vi "EncoderB(D0BD).vi"() -> ()   [LabVIEW 2021]
uses:
  BISS_1SL_interface_7.7.0/lv_interface/enum/BISS_InterfaceEnum.ctl
  BISS_1SL_interface_7.7.0/lv_interface/enum/BISS_InterfaceInfoEnum.ctl
  BISS_1SL_interface_7.7.0/lv_interface/enum/BISS_ComParamEnum.ctl
  BISS_1SL_interface_7.7.0/lv_interface/enum/BISS_FrameParamEnum.ctl
  BISS_1SL_interface_7.7.0/lv_interface/enum/BISS_EdsParamEnum.ctl
  BISS_1SL_interface_7.7.0/lv_interface/enum/BISS_ErrorTypeEnum.ctl
  BISS_1SL_interface_7.7.0/lv_interface/dll_demo/BiSS Interface Demo Functions.ctl
  BISS_1SL_interface_7.7.0/lv_interface/BISS1SL_Interface.lvlib
panel:
  in  "Stop Button":bool
  in  "TabControl":T1(tab)
  in  "BISS_InterfaceInfoEnum":T2 format="0x%02x"
  out "BISS_InterfaceEnum":T3 format="0x%02x"
  in  "BISS_InterfaceEnum":T3=enum."BISS_MB5U" format="0x%02x"
  in  "Close":bool caption="BiSS_Close"
  in  "Get Interface":bool caption="BiSS_GetInterface"
  in  "Set Interface":bool caption="BiSS_SetInterface"
  in  "Open":bool caption="BiSS_Open"
  in  "pcInterfaceOption":string="D0BD"
  in  "Get Interface Info":bool caption="BiSS_GetInterfaceInfo"
  out "pcInterfaceInfo":string
  in  "Write Master Params":bool caption="BiSS_WriteMasterParams"
  in  "pcFilename":path
  in  "Load DLL Config":bool caption="BiSS_LoadDLLConfig"
  in  "pcFilename 2":path=path "C:/Users/TSSW/Documents/Kenneth Feb/BISS Test Vi/BiSS_config.cfg"
  in  "Save DLL Config":bool caption="BiSS_SaveDLLConfig"
  in  "Get Slave Label":bool caption="BiSS_GetSlaveLabel"
  in  "ulSlave 2":u32 format="%.0x"
  out "pcCompleteLabel 2":string
  out "pcSlaveLabel 2":string
  out "pcManufacturerLabel 2":string
  in  "Set FTDI Freq":bool caption="BiSS_SetFTDIFreq"
  in  "ulFreqL":u32=4 format="%0x"
  in  "ulFreqH":u32=4 format="%0x"
  out "Displacement vs Time":waveform(sgl)(graph)
  out "pulValues":u64[](array[numeric]) format="%.0x"
  in  "ulCycleCount":u32 format="%.0x"
  in  "ulContentIndex":u32 format="%.0x"
  in  "ulDataChannel":u32 format="%.0x"
  in  "Get SCD Frame Content Ex":bool caption="BiSS_GetScdFrameContentEx"
  in  "Read SCD Frames":bool caption="BiSS_ReadScdFrames"
  in  "ulCycleCnt":u32=1 format="%.0x"
  out "pulDataScdH":u32[](array[numeric]) format="%.0x"
  out "pulDataScdL":sgl[](array[numeric]) format="%#_8g mm"
  out "pulStatus":u32[](array[numeric]) format="%.0x"
  out "pulTimestamp":u32[](array[numeric]) format="%.0x"
  in  "Get SCD Frame":bool caption="BiSS_GetScdFrame"
  in  "ulFrameIndex":u32 format="%.0x"
  out "pulDataScdH":u32[](array[numeric]) format="%.0x"
  out "pulDataScdL":u32[](array[numeric]) format="%.0x"
  out "pulStatus":u32 format="%.0x"
  out "pulTimestamp":u32 format="%.0x"
  in  "ulDataChannel":u32 format="%.0x"
  in  "Get SCD Frame Ex":bool caption="BiSS_GetScdFrameEx"
  in  "ulCycleCount":u32 format="%.0x"
  out "pulTimestamp":u32[](array[numeric]) format="%.0x"
  out "pulDataScdH":u32[](array[numeric]) format="%.0x"
  out "pulDataScdL":u32[](array[numeric]) format="%.0x"
  out "pulStatus":u32[](array[numeric]) format="%.0x"
  in  "Get SCD Frame Content":bool caption="BiSS_GetScdFrameContent"
  in  "ulDataChannel":u32 format="%.0x"
  in  "ulContentIndex":u32 format="%.0x"
  out "pulValues":u32[](array[numeric]) format="%.0x"
  in  "ulCycleCount":u32 format="%.0x"
  in  "stop":bool
  out "Loop Time [ms]":u32
  in  "Update Time [ms]":u32=1000
  out "BISS_ErrorTypeEnum":T4 format="0x%02x"
  in  "Get DLL Version":bool caption="BiSS_GetDLLVersion"
  out "pulDllVersion":u32[](array[numeric]) format="%.0x"
  in  "Calculate CRC":bool caption="BiSS_CalculateCRC"
  in  "ulCrcPoly":u32 format="%.0x"
  in  "pulData":u32[](array[numeric]) format="%.0x"
  in  "ulByteCount":u32 format="%.0x"
  out "pulCheckSum":u32 format="%.0x"
  in  "Calculate CRC Ex":bool caption="BiSS_CalculateCRCEx"
  out "pulCheckSum":u32 format="%.0x"
  in  "ulByteCount":u32 format="%.0x"
  in  "pulData":u32[](array[numeric]) format="%.0x"
  in  "ulCrcPoly":u32 format="%.0x"
  in  "ulCRCStartValue":u32 format="%.0x"
  in  "Get Last Error":bool caption="BiSS_GetLastError"
  out "pulLastError":u32 format="%0x"
  out "pcErrorText":string
  in  "Get MB3U Pins":bool caption="BiSS_GetMB3UPins"
  out "pulDir":u32 format="%.0x"
  out "pulValue":u32 format="%.0x"
  in  "ulDir":u32 format="%.0x"
  in  "Set MB3U Pins":bool caption="BiSS_SetMB3UPins"
  in  "ulValue":u32 format="%.0x"
  in  "Set Slave Label":bool caption="BiSS_SetSlaveLabel"
  in  "ulSlave":u32 format="%.0x"
  in  "pcSlaveLabel":string
  in  "pcManufacturerLabel":string
  in  "pcCompleteLabel":string
  in  "Set SCD Content Labels":bool caption="BiSS_SetScdContentLabels"
  in  "ulDataChannel":u32 format="%.0x"
  in  "ulContentIndex":u32 format="%.0x"
  in  "pcScdContentLabel":string
  in  "pcScdContentUnit":string
  in  "Get SCD Content Labels":bool caption="BiSS_GetScdContentLabels"
  in  "ulDataChannel":u32 format="%.0x"
  in  "ulContentIndex":u32 format="%.0x"
  out "pcSCDContentLabel":string
  out "pcSCDContentUnit":string
  in  "BISS_FrameParamEnum":T5 format="0x%02x"
  in  "BISS_FrameParamEnum":T5 format="0x%02x"
  in  "BISS_ComParamEnum":T6 format="0x%02x"
  in  "BISS_ComParamEnum":T6 format="0x%02x"
  in  "pcFilename":path
  in  "Set Com Param":bool caption="BiSS_SetComParam"
  in  "Auto Detection":bool caption="BiSS_Autodetection"
  in  "ulWriteMasterParams":u32 format="%.0x"
  out "pulSlaveCount":u32 format="%.0x"
  in  "ulValue":u32 format="%.0x"
  in  "Get Com Param":bool caption="BiSS_GetComParam"
  out "pulValue":u32 format="%.0x"
  in  "Set Frame Param":bool caption="BiSS_FrameParamEnum"
  in  "ulDataChannel":u32 format="%.0x"
  in  "ulValue":u32 format="%.0x"
  in  "Get Frame Param":bool caption="BiSS_GetFrameParam"
  out "pulValue":u32 format="%.0x"
  in  "ulDataChannel":u32 format="%.0x"
  in  "Init BiSS Comm":bool caption="BiSS_InitBissComm"
  in  "Write Slave Register":bool caption="BiSS_WriteSlaveRegister"
  in  "ulProtocol":u32 format="%.0x"
  in  "ulSlaveId":u32 format="%.0x"
  in  "ulRegisterAddress":u32 format="%.0x"
  in  "pulRegisterContent":u32[](array[numeric]) format="%.0x"
  in  "pulNumberOfBytes":u32 format="%.0x"
  in  "Read Slave Register":bool caption="BiSS_ReadSlaveRegister"
  in  "ulProtocol":u32 format="%.0x"
  in  "ulSlaveId":u32 format="%.0x"
  in  "ulRegisterAddress":u32 format="%.0x"
  in  "pulNumberOfBytes":u32 format="%.0x"
  out "pulRegisterContent":u32[](array[numeric]) format="%.0x"
  in  "Read SCD":bool caption="BiSS_ReadSCD"
  in  "ulStartControlFrame":u32 format="%.0x"
  out "pulScdValid":u32 format="%.0x"
  out "pulControlFrameEnd":u32 format="%.0x"
  out "pulDataScdH":u32[](array[numeric]) format="%.0x"
  out "pulDataScdL":u32[](array[numeric]) format="%.0x"
  in  "ulIds":u32 format="%.0x"
  in  "ulCmd":u32 format="%.0x"
  in  "Send Command":bool caption="BiSS_SendCommand"
  in  "Get SCD Content":bool caption="BiSS_GetScdContent"
  in  "ulDataChannel":u32 format="%.0x"
  out "pulScdContentValues":u32[](array[numeric]) format="%.0x"
  in  "Get SCD Content Ex":bool caption="BiSS_GetScdContentEx"
  in  "ulDataChannel":u32 format="%.0x"
  out "pulScdContentValues":u64[](array[numeric]) format="%.0x"
  in  "Set SCD Content Params":bool caption="BiSS_SetScdContentParams"
  in  "ulDataChannel":u32 format="%.0x"
  in  "ulContentIndex":u32 format="%.0x"
  in  "pScdContentItems":T7 {"lOffset" format="%.0x"; "ulResolution" format="%.0x"; "ulDataLength" format="%.0x"; "ulZero" format="%.0x"}
  in  "Get SCD Content Params":bool caption="BiSS_GetScdContentParams"
  in  "ulDataChannel":u32 format="%.0x"
  in  "ulContentIndex":u32 format="%.0x"
  out "pScdContentItems":T7 {"ulZero" format="%.0x"; "ulDataLength" format="%.0x"; "ulResolution" format="%.0x"; "lOffset" format="%.0x"}
  in  "BISS_EdsParamEnum":T8 format="0x%02x"
  in  "BISS_EdsParamEnum":T8 format="0x%02x"
  in  "Set EDS Param":bool caption="BiSS_SetEdsParam"
  in  "ulValue":u32 format="%.0x"
  out "pulValue":u32 format="%.0x"
  in  "Get EDS Param":bool caption="BiSS_GetEdsParam"
  in  "Set EDS Register":bool caption="BiSS_SetEdsRegister"
  in  "ulAdr":u32 format="%.0x"
  in  "ulValue":u32 format="%.0x"
  in  "Get EDS Register":bool caption="BiSS_GetEdsRegister"
  in  "ulAdr":u32 format="%.0x"
  out "pulValue":u32 format="%.0x"
  in  "Read EDS Params":bool caption="BiSS_ReadEdsParams"
  in  "ulSlaveId":u32 format="%.0x"
  in  "Write EDS Params":bool caption="BiSS_WriteEdsParams"
  in  "ulSlaveId":u32 format="%.0x"
  in  "pcFilename":path
  in  "Write Master Register":bool caption="BiSS_ WriteMasterRegister"
  in  "ulRegisterAddress":u32 format="%.0x"
  in  "ulRegisterContent":u32 format="%.0x"
  in  "Read Master Register":bool caption="BiSS_ ReadMasterRegister"
  in  "ulRegisterAddress":u32 format="%.0x"
  out "pulRegisterContent":u32 format="%.0x"
  in  "Get Master Register":bool caption="BiSS_ GetMasterRegister"
  in  "ulRegisterAddress":u32 format="%.0x"
  out "pulRegisterContent":u32 format="%.0x"
  in  "Save Master Config":bool caption="BiSS_ SaveMasterConfig"
  in  "pcFilename":path
  in  "Save Register":bool caption="BiSS_ SaveRegister"
  in  "pcFilename":path
  in  "ulStartAdr":u32 format="%.0x"
  in  "ulNumberOfBytes":u32 format="%.0x"
  in  "pulData":u32[](array[numeric]) format="%.0x"
  in  "Load Register":bool caption="BiSS_ LoadRegister"
  in  "ulStartAdr":u32 format="%.0x"
  in  "ulNumberOfBytes":u32 format="%.0x"
  out "pulData":u32[](array[numeric]) format="%.0x"
  # "BiSS Interface Library Demo"
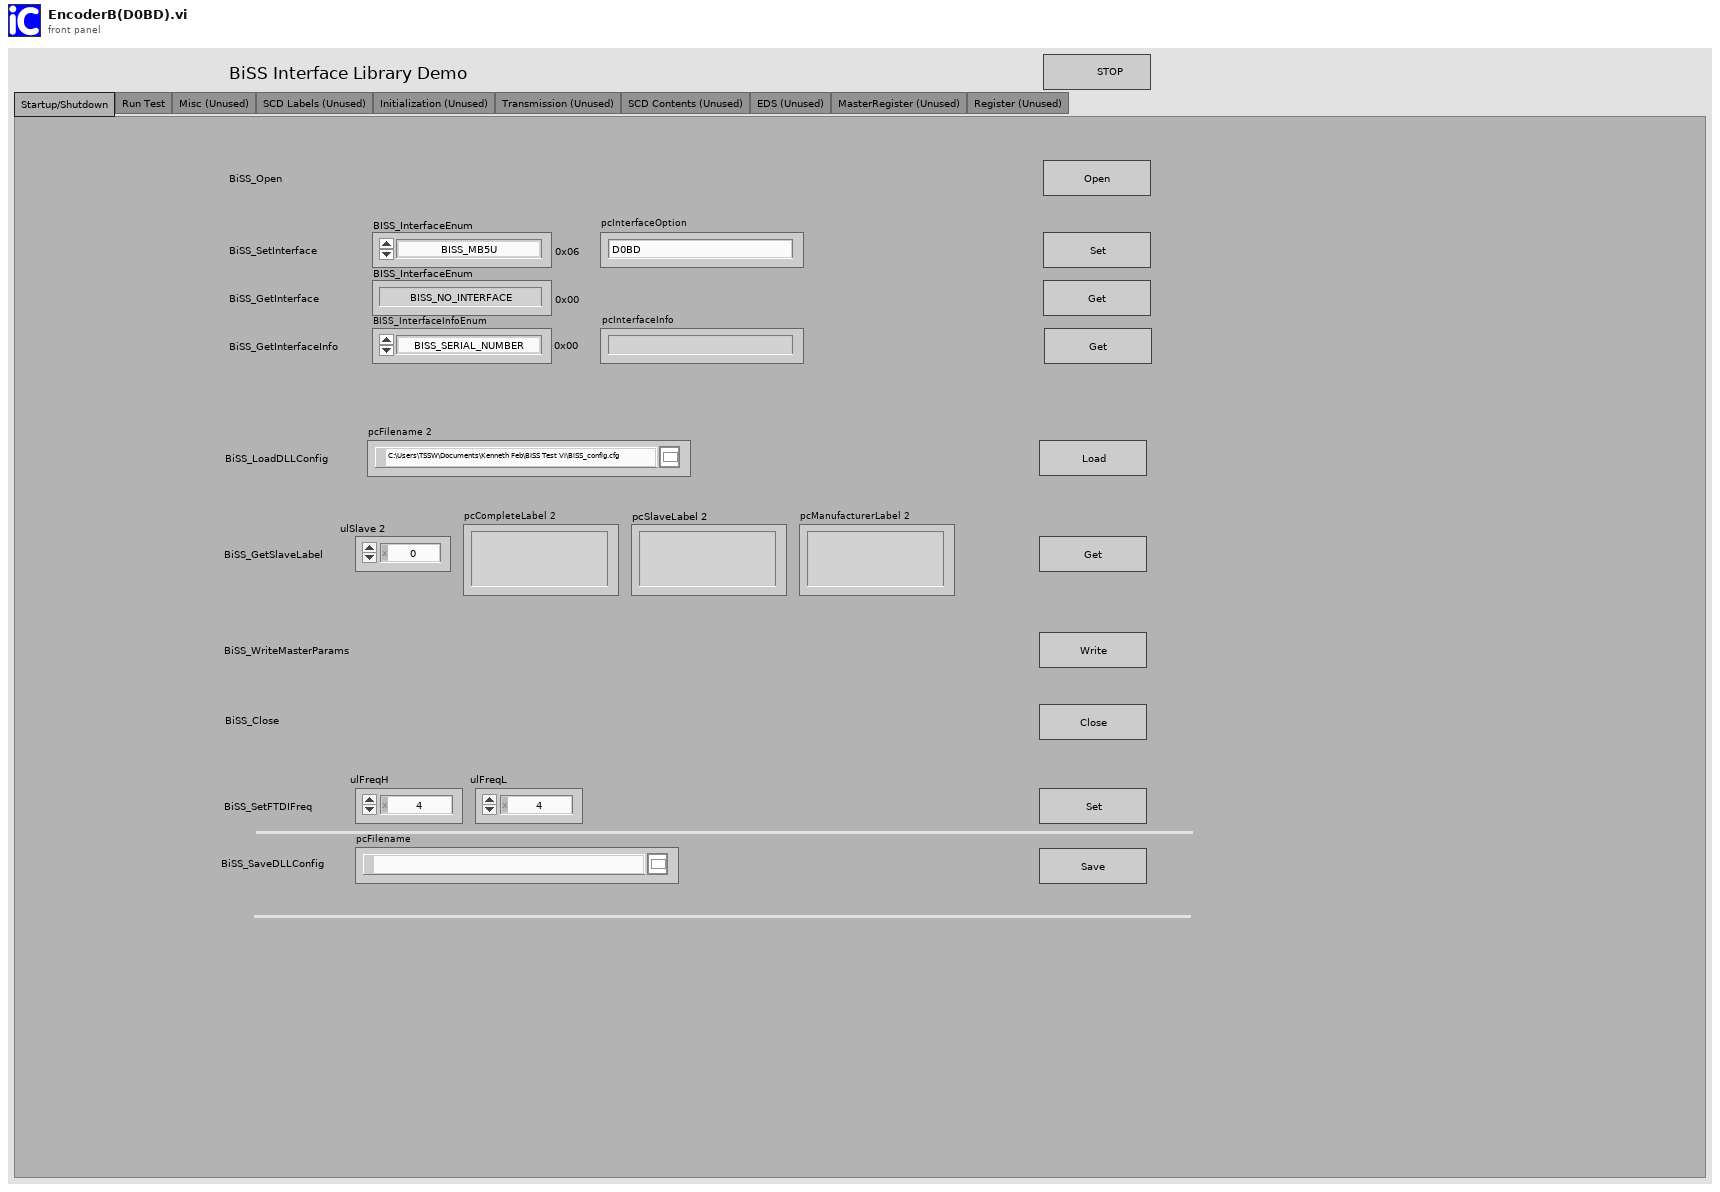
[diagram p1: front panel]
types:
  T1 = enum32{"Startup/Shutdown", "Run Test", "Misc (Unused)", "SCD Labels (Unused)", "Initialization (Unused)", "Transmission (Unused)", "SCD Contents (Unused)", "EDS (Unused)", "MasterRegister (Unused)", "Register (Unused)"}
  T2 = typedef "BISS1SL_Interface.lvlib/BISS_InterfaceInfoEnum.ctl" = enum32{"BISS_SERIAL_NUMBER", "BISS_DRIVER_VERSION"}
  T3 = typedef "BISS1SL_Interface.lvlib/BISS_InterfaceEnum.ctl" = enum32{"BISS_NO_INTERFACE", "BISS_MB3D_INT", "BISS_MB3D_MOT", "BISS_MB3A", "BISS_MB3U", "BISS_MB4U", "BISS_MB5U", "BISS_MB3U_SPI"}
  T4 = typedef "BISS1SL_Interface.lvlib/BISS_ErrorTypeEnum.ctl" = enum32{"BISS_NONE", "BISS_HINT", "BISS_WARNING", "BISS_PROGRAMMING_ERROR", "BISS_OPERATING_ERROR", "BISS_COMMUNICATION_ERROR"}
  T5 = typedef "BISS1SL_Interface.lvlib/BISS_FrameParamEnum.ctl" = enum32{"BISS_SCD_LENGTH", "BISS_SCD_CRC_POLY", "BISS_SCD_CRC_INVERT", "BISS_SCD_CONTENT_COUNT", "BISS_RESERVED", "BISS_SLAVEID", "BISS_IDCOUNT", "BISS_CRCS", "BISS_GRAYS", "BISS_GRAY_MSB", "BISS_GRAY_LSB", "BISS_CRC_CLOSING_VALUE"}
  T6 = typedef "BISS1SL_Interface.lvlib/BISS_ComParamEnum.ctl" = enum32{"BISS_MASTER_VERSION", "BISS_MASTER_REVISION", "BISS_PROTOCOL", "BISS_CLKENI", "BISS_FREQ_SCD", "BISS_FREQ_REG", "BISS_FREQ_AGS", "BISS_SLAVE_ID", "BISS_REGISTER_ADDRESS", "BISS_WNR", "BISS_REGISTER_VALUE", "BISS_SSIWRITE", "BISS_SSIWRITE_TIMEOUT", "BISS_MAX_DATACH_CNT", "BISS_MAX_REG_CNT", "BISS_EN_MO", "BISS_FREQ_AGS_REG", "BISS_EDS_BANK", "BISS_DISABLE_TIMEOUT", "BISS_ENABLE_TTL", "BISS_NUMBER_OF_DATA_CHANNELS", "BISS_SSIWRITE_DL", "BISS_SLAVELOC"}
  T7 = cluster{"ulZero":u32, "ulDataLength":u32, "ulResolution":u32, "lOffset":i32}
  T8 = typedef "BISS1SL_Interface.lvlib/BISS_EdsParamEnum.ctl" = enum32{"BISS_EDS_EDS_VER", "BISS_EDS_EDS_LEN", "BISS_EDS_USR_STA", "BISS_EDS_USR_END", "BISS_EDS_TMA", "BISS_EDS_TO_MIN", "BISS_EDS_TO_MAX", "BISS_EDS_TOS_MIN", "BISS_EDS_TOS_MAX", "BISS_EDS_TCLK_MIN", "BISS_EDS_TCLK_MAX", "BISS_EDS_TCYC", "BISS_EDS_TBUSY_S", "BISS_EDS_BUSY_S", "BISS_EDS_PON_DLY", "BISS_EDS_DC_NUM", "BISS_EDS_SL_NUM", "BISS_EDS_SL_OFF", "BISS_EDS_BANK1", "BISS_EDS_DLEN1", "BISS_EDS_FORMAT1_STOP", "BISS_EDS_FORMAT1_ALIGN", "BISS_EDS_FORMAT1_TYPE", "BISS_EDS_CPOLY1", "BISS_EDS_BANK2", "BISS_EDS_DLEN2", "BISS_EDS_FORMAT2_STOP", "BISS_EDS_FORMAT2_ALIGN", "BISS_EDS_FORMAT2_TYPE", "BISS_EDS_CPOLY2", "BISS_EDS_BANK3", "BISS_EDS_DLEN3", "BISS_EDS_FORMAT3_STOP", "BISS_EDS_FORMAT3_ALIGN", "BISS_EDS_FORMAT3_TYPE", "BISS_EDS_CPOLY3", "BISS_EDS_BANK4", "BISS_EDS_DLEN4", "BISS_EDS_FORMAT4_STOP", "BISS_EDS_FORMAT4_ALIGN", "BISS_EDS_FORMAT4_TYPE", "BISS_EDS_CPOLY4", "BISS_EDS_BANK5", "BISS_EDS_DLEN5", "BISS_EDS_FORMAT5_STOP", "BISS_EDS_FORMAT5_ALIGN", "BISS_EDS_FORMAT5_TYPE", "BISS_EDS_CPOLY5", "BISS_EDS_BANK6", "BISS_EDS_DLEN6", "BISS_EDS_FORMAT6_STOP", "BISS_EDS_FORMAT6_ALIGN", "BISS_EDS_FORMAT6_TYPE", "BISS_EDS_CPOLY6", "BISS_EDS_BANK7", "BISS_EDS_DLEN7", "BISS_EDS_FORMAT7_STOP", "BISS_EDS_FORMAT7_ALIGN", "BISS_EDS_FORMAT7_TYPE", "BISS_EDS_CPOLY7", "BISS_EDS_BANK8", "BISS_EDS_DLEN8", "BISS_EDS_FORMAT8_STOP", "BISS_EDS_FORMAT8_ALIGN", "BISS_EDS_FORMAT8_TYPE", "BISS_EDS_CPOLY8", "BISS_EDS_BC_OFF", "BISS_EDS_BP_VER", "BISS_EDS_BP_LEN", "BISS_EDS_BP_ID", "BISS_EDS_FB1", "BISS_EDS_FB2", "BISS_EDS_PON_PDL", "BISS_EDS_EN_TYP", "BISS_EDS_POS_NUM", "BISS_EDS_MT_LEN", "BISS_EDS_MT_FMT", "BISS_EDS_CO_LEN", "BISS_EDS_CO_FMT", "BISS_EDS_FI_LEN", "BISS_EDS_FI_FMT", "BISS_EDS_MT_CNT", "BISS_EDS_SIP_CNT", "BISS_EDS_SIP_RES", "BISS_EDS_CPOLY", "BISS_EDS_CSTART", "BISS_EDS_ABS_ACU", "BISS_EDS_REL_ACU", "BISS_EDS_SPD_ACU", "BISS_EDS_HYST", "BISS_EDS_SPD_MAX", "BISS_EDS_ACC_MAX", "BISS_EDS_TMP_MIN", "BISS_EDS_TMP_MAX", "BISS_EDS_VLT_MIN", "BISS_EDS_VLT_MAX", "BISS_EDS_CUR_MAX"}
  T9 = typedef "BiSS Interface Demo Functions.ctl" = enum16{"Start Demo", "Open", "Close", "Set Interface", "Set Interface 2", "Get Interface", "Get Interface 2", "Get Interface Info", "Get Interface Info 2", "Auto Detection", "Set Com Param", "Get Com Param", "Set Frame Param", "Get Frame Param", "Write Master Params", "Set FTDI Freq", "Init BiSS Comm", "Write Slave Register", "Read Slave Register", "Read SCD", "Send Command", "Set Slave Label", "Get Slave Label", "Set SCD Content Labels", "Get SCD Content Labels", "Get SCD Content", "Get SCD Content Ex", "Set SCD Content Params", "Get SCD Content Params", "Read SCD Frames", "Get SCD Frame", "Get SCD Frame Ex", "Get SCD Frame Content", "Get SCD Frame Content Ex", "Set EDS Param", "Get EDS Param", "Set EDS Register", "Get EDS Register", "Read EDS Params", "Write EDS Params", "Get DLL Version", "Calculate CRC", "Calculate CRC Ex", "Save DLL Config", "Load DLL Config", "Get Last Error", "Get MB3U Pins", "Set MB3U Pins", "Write Master Register", "Read Master Register", "Get Master Register", "Save Master Config", "Save Register", "Load Register", "Stop Demo"}
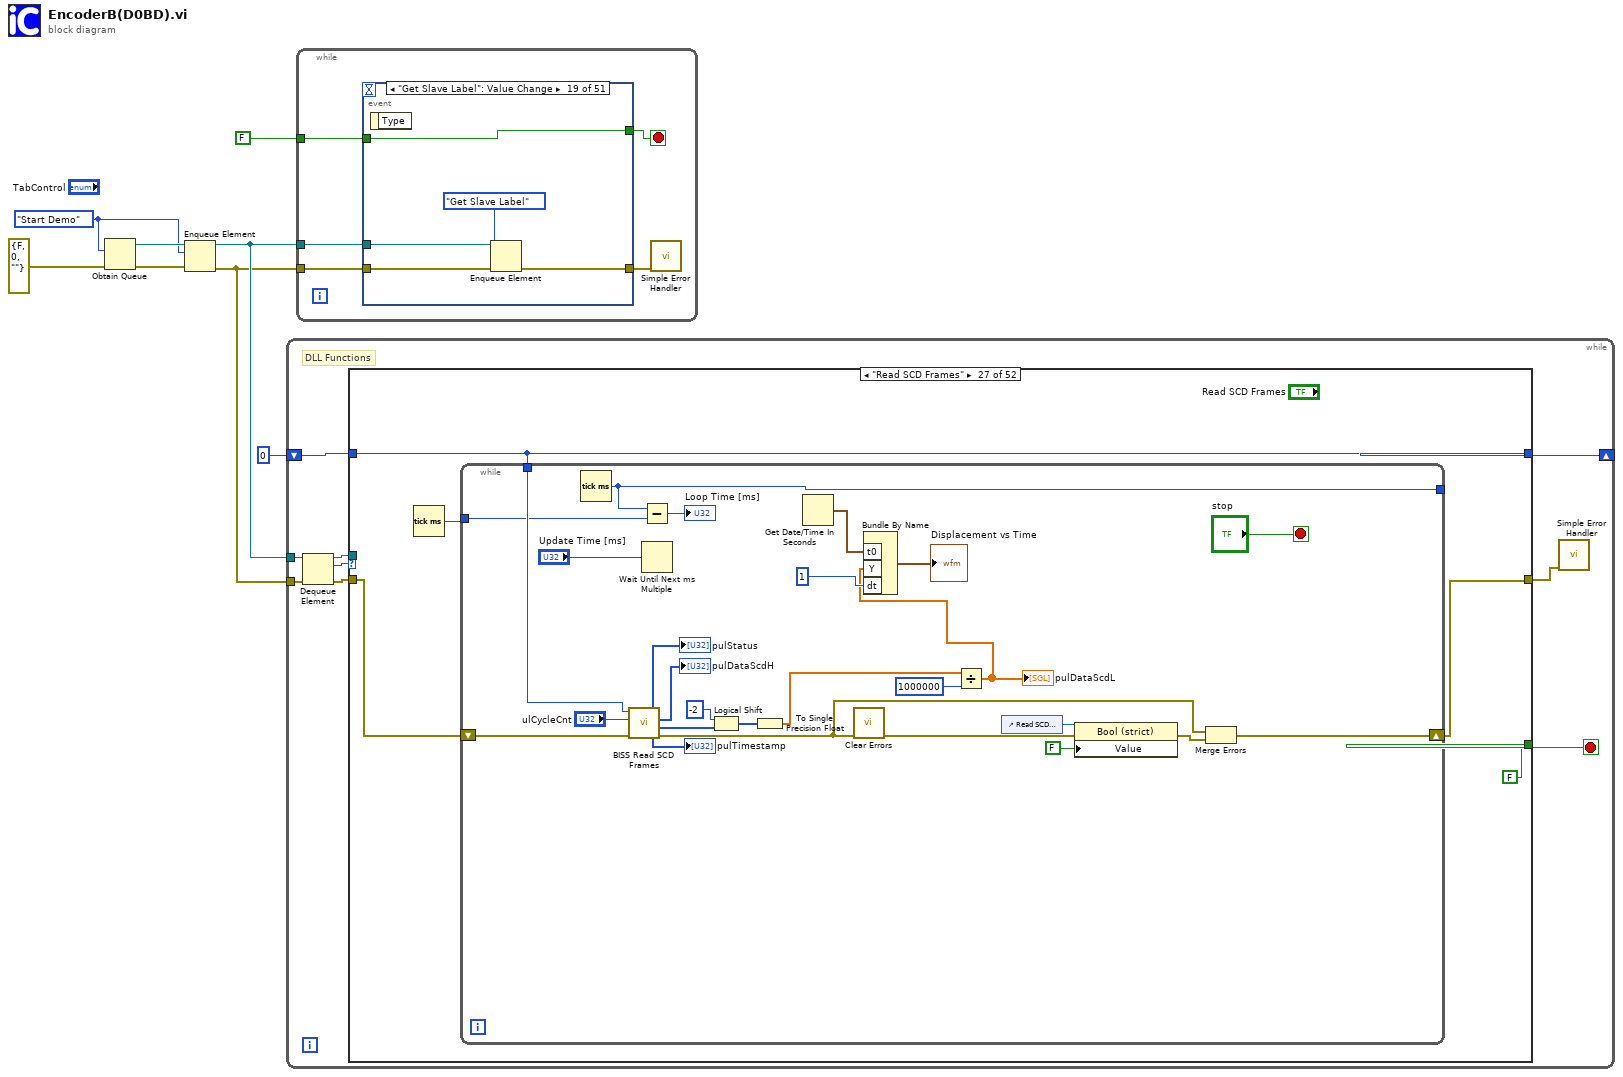
[diagram p0: block diagram]
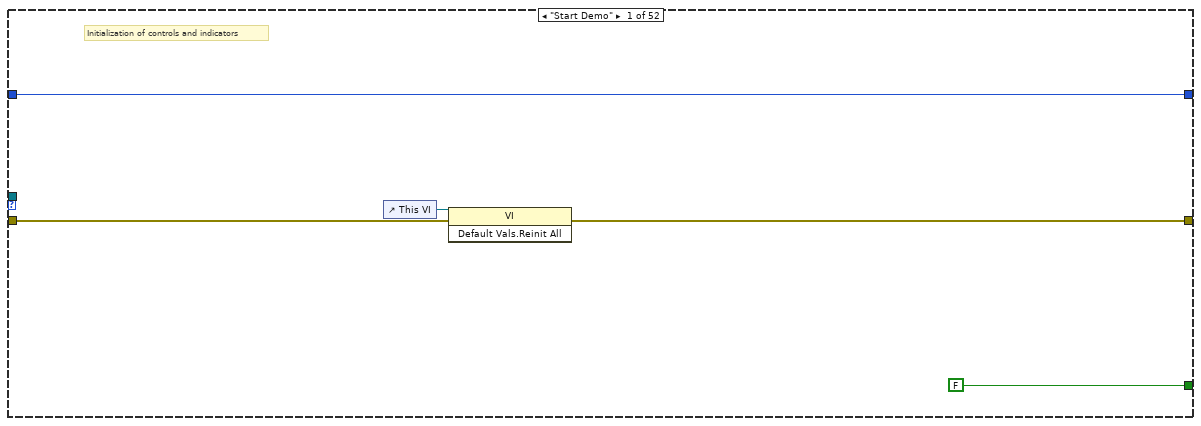
[diagram p2: hidden frame]
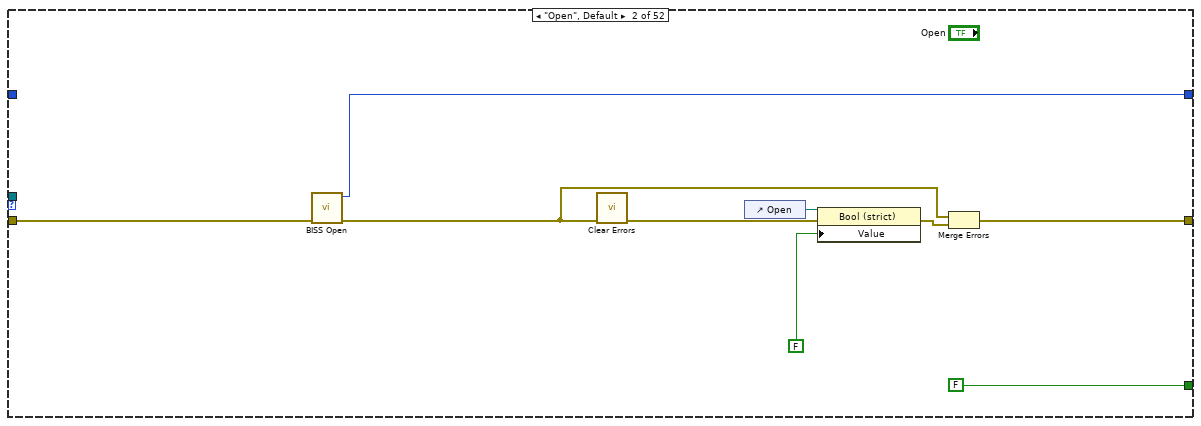
[diagram p3: hidden frame]
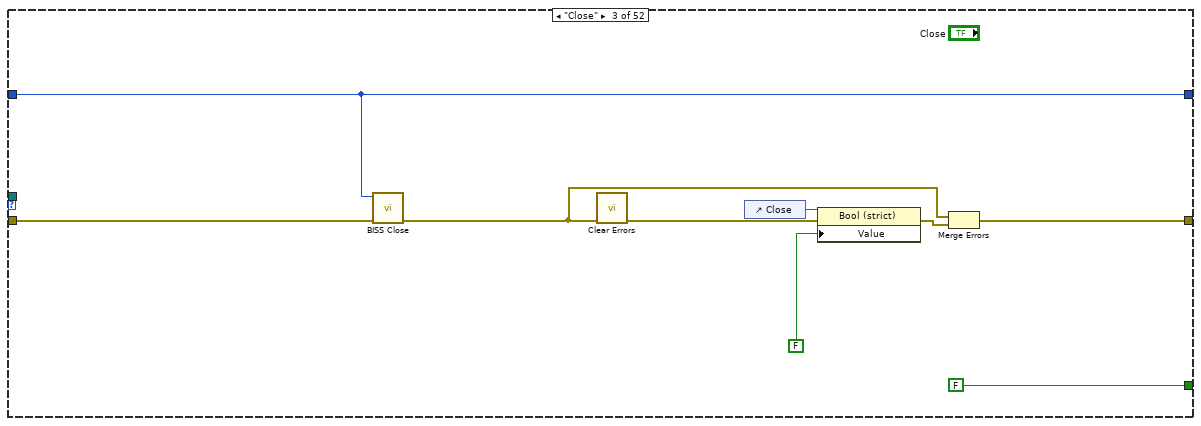
[diagram p4: hidden frame]
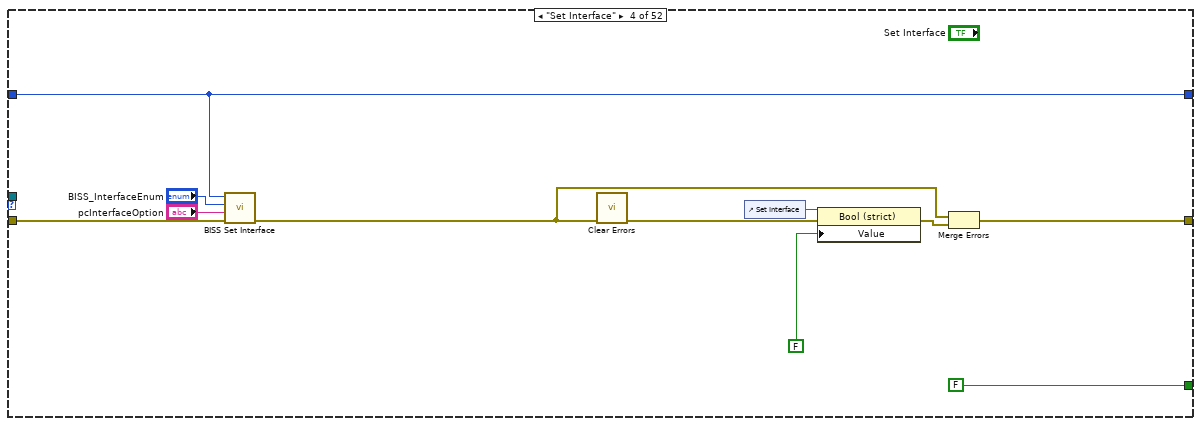
[diagram p5: hidden frame]
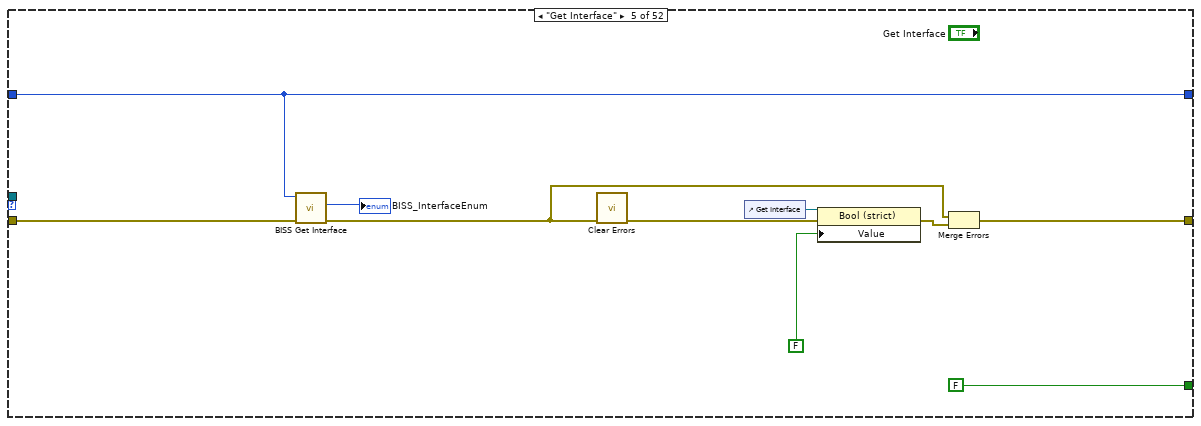
[diagram p6: hidden frame]
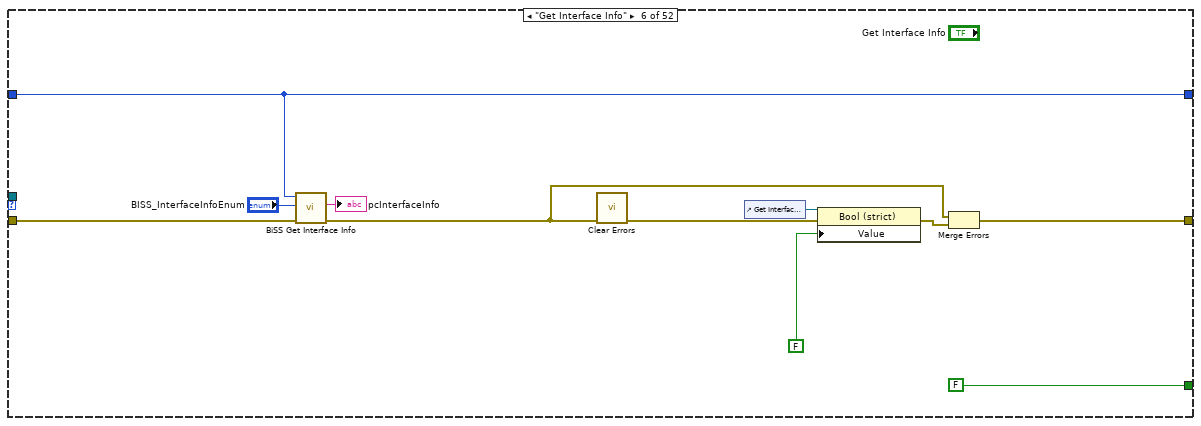
[diagram p7: hidden frame]
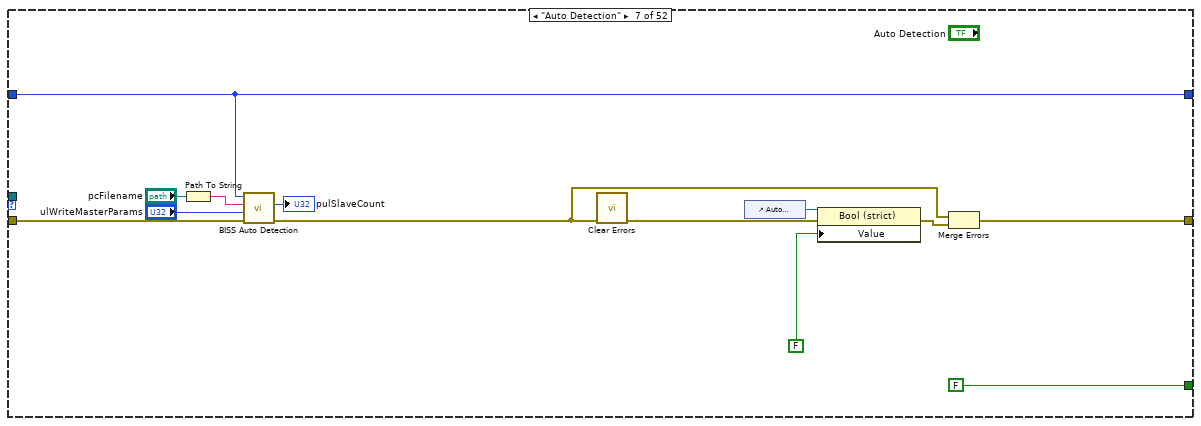
[diagram p8: hidden frame]
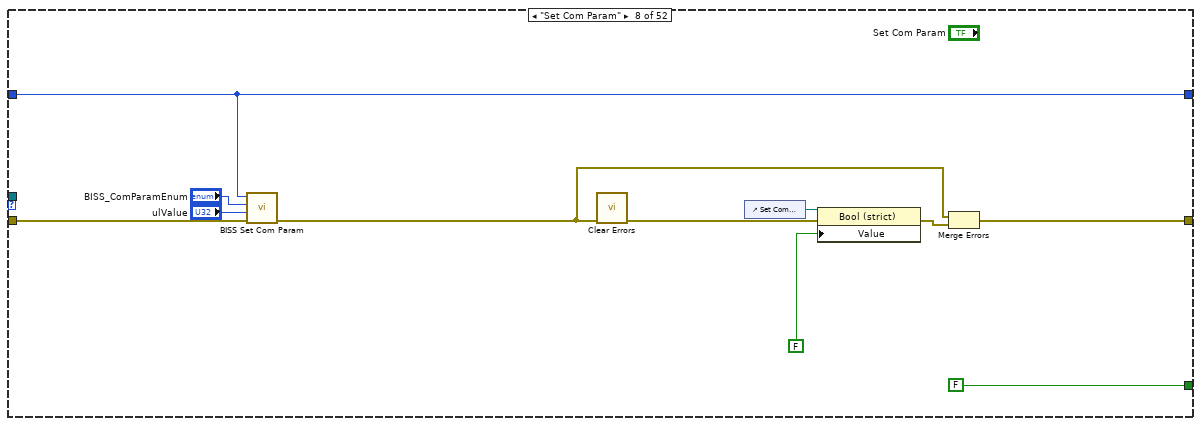
[diagram p9: hidden frame]
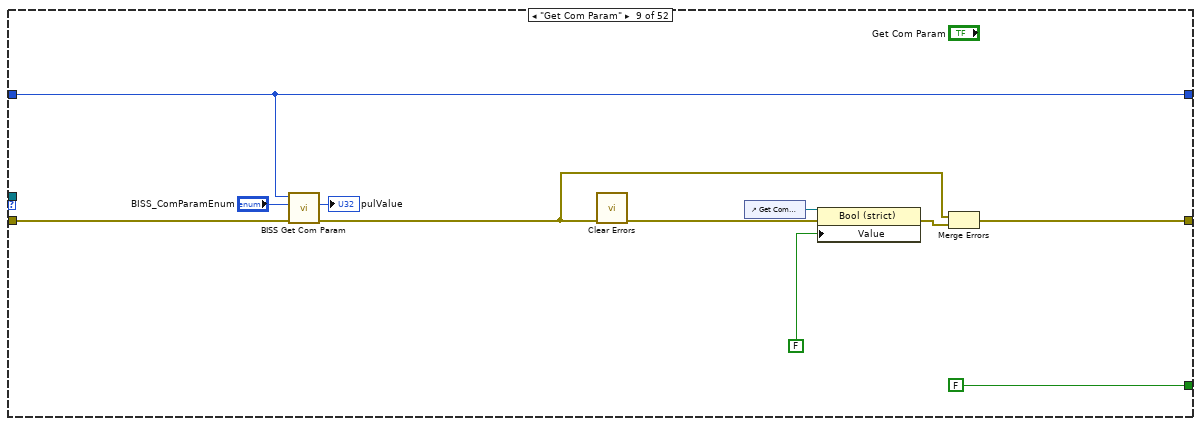
[diagram p10: hidden frame]
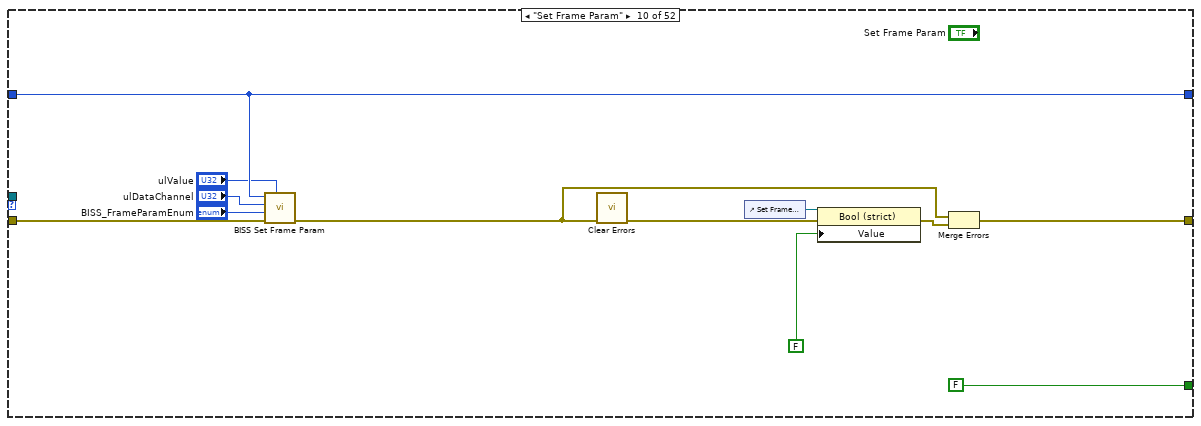
[diagram p11: hidden frame]
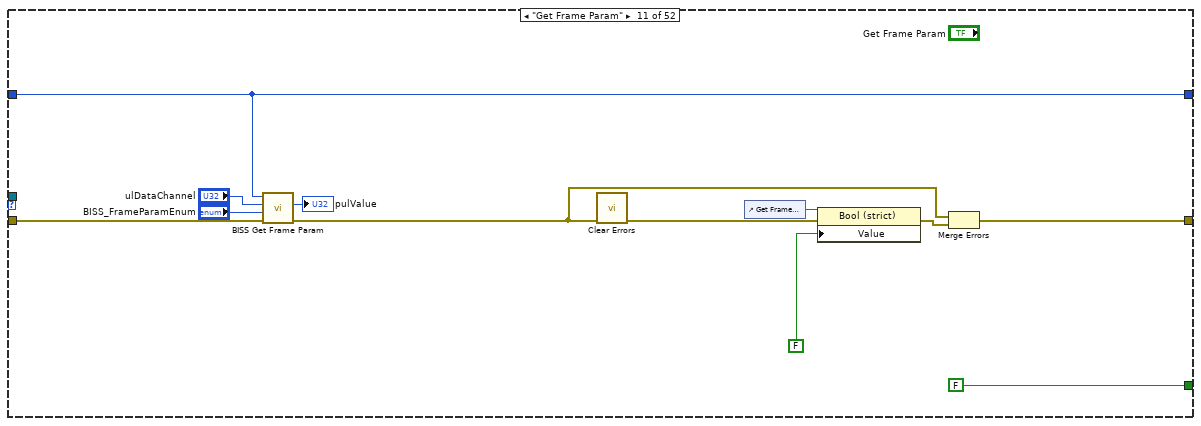
[diagram p12: hidden frame]
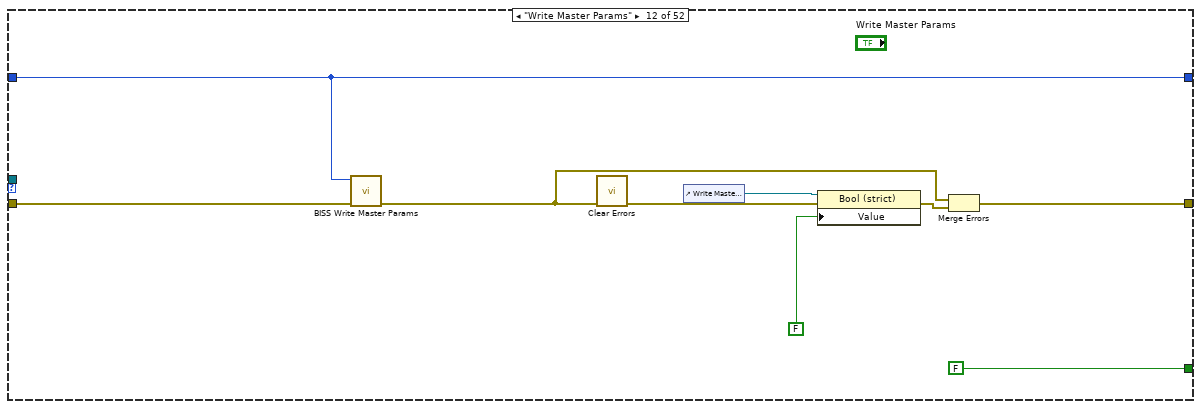
[diagram p13: hidden frame]
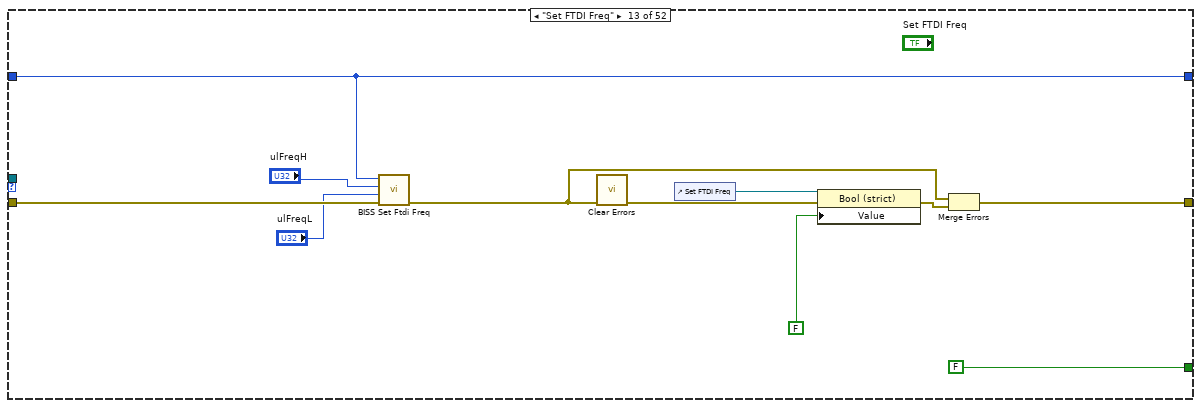
[diagram p14: hidden frame]
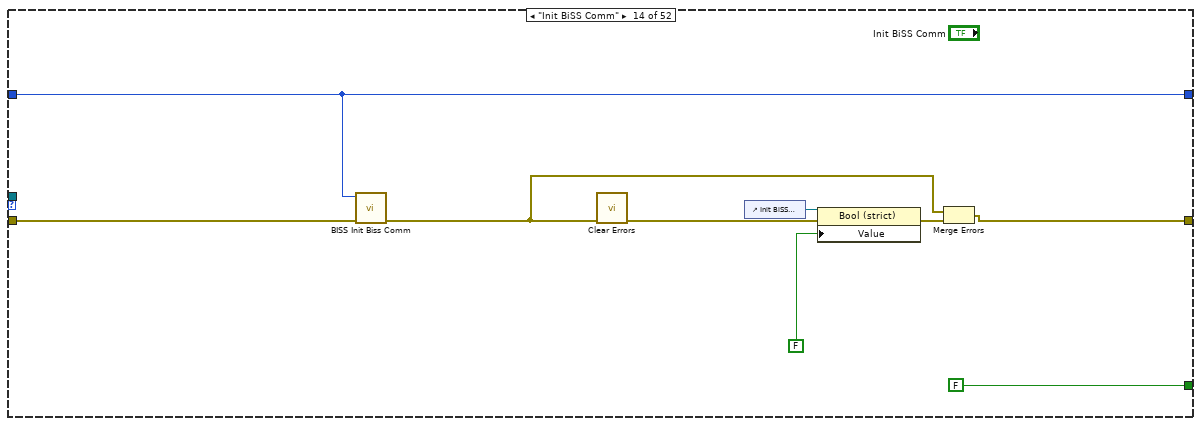
[diagram p15: hidden frame]
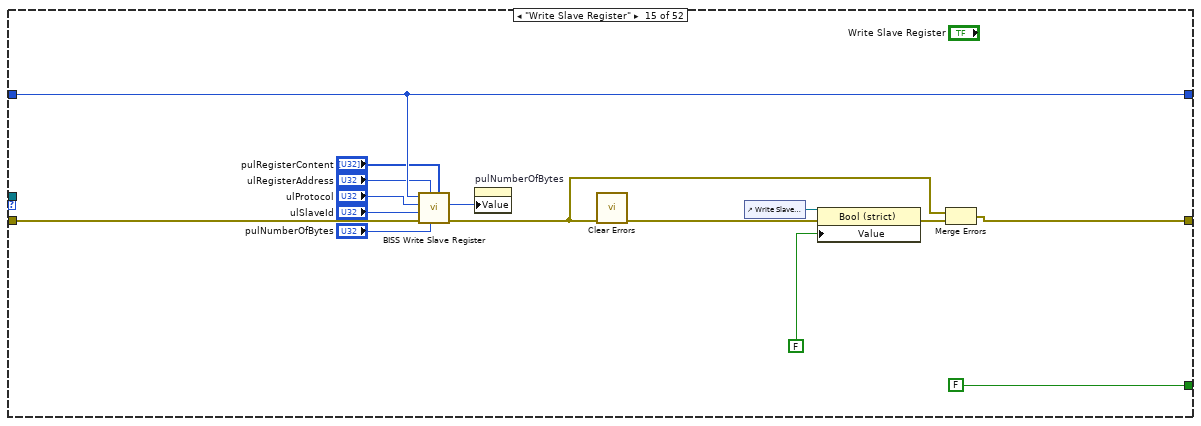
[diagram p16: hidden frame]
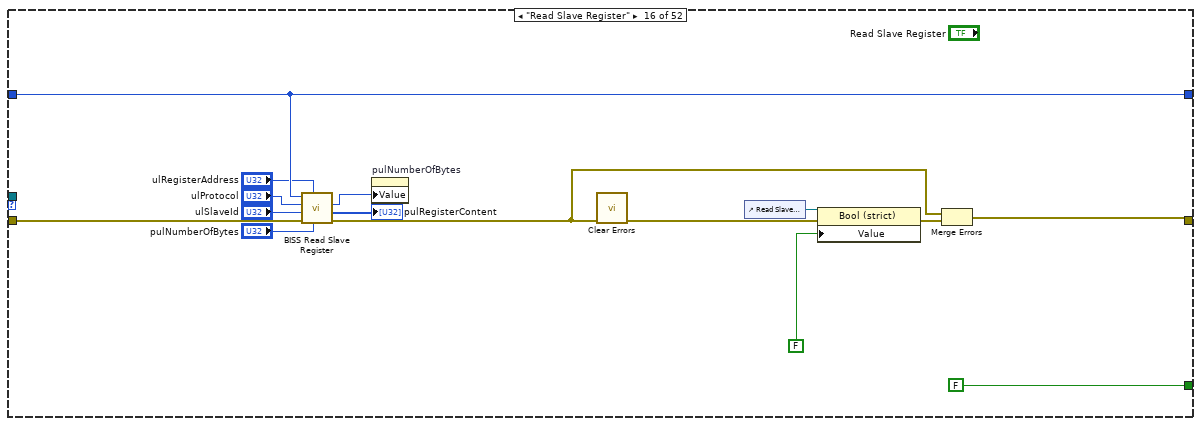
[diagram p17: hidden frame]
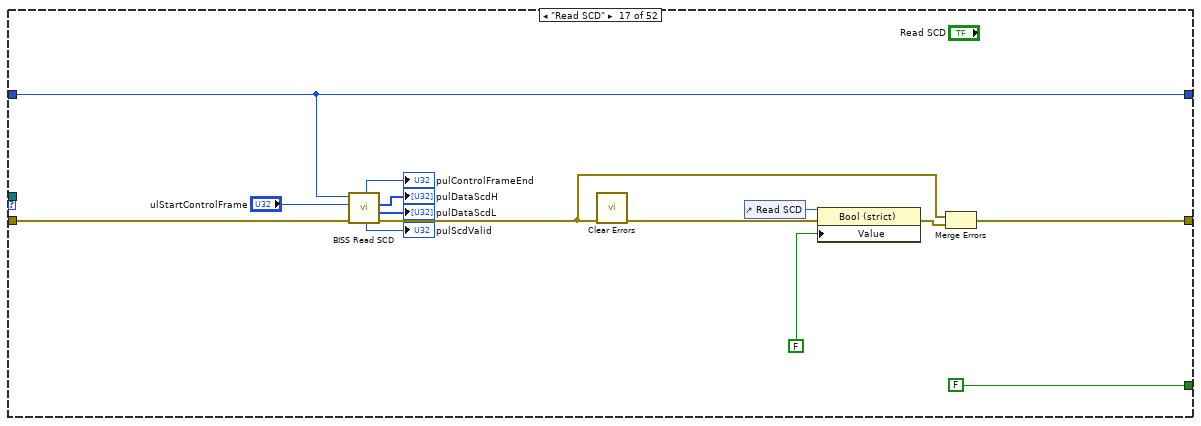
[diagram p18: hidden frame]
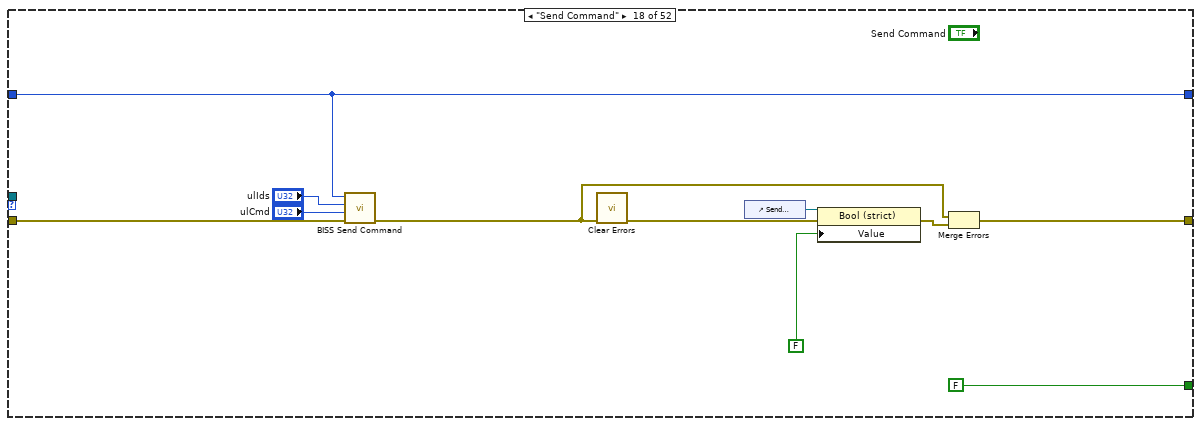
[diagram p19: hidden frame]
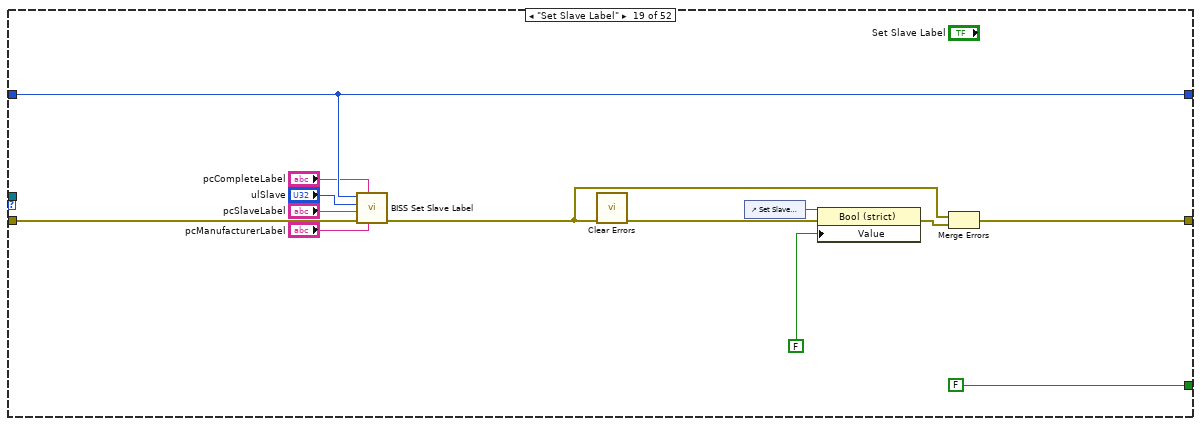
[diagram p20: hidden frame]
diagram:
  w2 = BiSS_Interface_Demo_Functions."Start Demo" ("Events")
  n1 = Obtain Queue(element data type=w2, error in (no error)=errorcluster {"status"=FALSE, "code"=0, "source"=""} ("error in")) -> (queue out=w7:refnum<queue>, error out=w8:errorcluster)  [unwired: 3 in, 1 out]
  n2 = Enqueue Element(queue=w7, element=w2, error in (no error)=w8) -> (queue out=w4:refnum<queue>, error out=w3:errorcluster)  [unwired: 1 in, 1 out]
  n3 = while {
    shift-right: [w15] -> _
    shift-left: u32 0 ("pulHTHandle") -> [w14]
    tunnel: w4 -> [w16]
    tunnel: w3 -> [w11]
    stop <- w12 stop-if-true
    # "DLL Functions"
    n4 = Dequeue Element(queue=w16, error in (no error)=w11) -> (queue out=w10:refnum<queue>, element=w17:T9, error out=w9:errorcluster)  [unwired: 1 in, 1 out]
    n5 = case shown="\"Read SCD Frames\"" w17 {
      tunnel: [w18 w26 w36 w47 w57 w68 w82 w93 w104 w116 w128 w138 w147 w152 w170 w182 w200 w210 w224 w239 w250 w263 w274 w285 w297 w309 w315 w354 w369 w382 w388 w405 w416 w427 w438 w448 w458 w468 w481 w495 w507 w518 w529 w540 w551 w562 w573 w584 w595 w609 w623 w634] -> w13
      tunnel: [FALSE FALSE FALSE FALSE FALSE FALSE FALSE FALSE FALSE FALSE FALSE FALSE FALSE FALSE FALSE FALSE FALSE FALSE FALSE FALSE FALSE FALSE FALSE FALSE FALSE FALSE FALSE FALSE FALSE FALSE FALSE FALSE FALSE FALSE FALSE FALSE FALSE FALSE FALSE FALSE FALSE FALSE FALSE FALSE FALSE FALSE FALSE FALSE FALSE FALSE FALSE TRUE] -> w12
      tunnel: [w22 w23 w33 w44 w53 w64 w78 w89 w101 w112 w124 w133 w144 w155 w167 w185 w196 w209 w221 w236 w246 w259 w270 w281 w293 w305 w316 w352 w365 w378 w397 w402 w413 w426 w437 w445 w455 w467 w478 w492 w506 w517 w526 w537 w548 w559 w570 w581 w592 w606 w620 w638] -> w15
      tunnel: w14 -> [w22 _ w33 w44 w53 w64 w78 w89 w101 w112 w124 w133 w144 w155 w167 w185 w196 w209 w221 w236 w246 w259 w270 w281 w293 w305 w316 w352 w365 w378 w397 w402 w413 w426 w437 w445 w455 w467 w478 w492 w506 w517 w526 w537 w548 w559 w570 w581 w592 w606 w620 w638]
      tunnel: w10 -> [_ _ _ _ _ _ _ _ _ _ _ _ _ _ _ _ _ _ _ _ _ _ _ _ _ _ _ _ _ _ _ _ _ _ _ _ _ _ _ _ _ _ _ _ _ _ _ _ _ _ _ w635]
      tunnel: w9 -> [w19 w25 w34 w45 w55 w66 w79 w90 w100 w113 w125 w135 w146 w156 w169 w184 w198 w208 w222 w235 w248 w261 w272 w283 w295 w307 w317 w351 w367 w380 w398 w404 w415 w425 w436 w447 w457 w466 w480 w494 w505 w516 w528 w539 w550 w561 w572 w583 w594 w608 w622 w636]
      frame "Start Demo" {
        # "Initialization of controls and indicators"
        n6 = control-ref of="This VI"() -> (w20:refnum<vi>)
        n7 = invoke class="VI" method="Default Vals.Reinit All"(reference=w20, error in=w19) -> (error out=w18:errorcluster)  [unwired: 1 in, 2 out]
      }
      frame "Open", Default {
        n8 = call "BISS Open.vi"("Error In"=w25) -> ("Error Out"=w24:errorcluster, "pulBISSHandle"=w23:u32)  [unwired: 7 in, 2 out]
        n9 = call <vilib>:"Clear Errors.vi"("error in (no error)"=w24) -> ("error out"=w28:errorcluster)  [unwired: 5 in, 1 out]
        n10 = control-ref of="Open"() -> (w30:refnum<vi>)
        n11 = property class="Bool (strict)"(reference=w30, error in=w28, "Value"=FALSE) -> (error out=w27:errorcluster)  [unwired: 1 out]
        n12 = Merge Errors(w24, w27) -> (w26:errorcluster)
      }
      frame "Close" {
        n13 = call "BISS Close.vi"("Error In"=w34, "ulBISSHandle"=w33) -> ("Error Out"=w32:errorcluster)  [unwired: 7 in, 2 out]
        n14 = call <vilib>:"Clear Errors.vi"("error in (no error)"=w32) -> ("error out"=w35:errorcluster)  [unwired: 5 in, 1 out]
        n15 = control-ref of="Close"() -> (w38:refnum<vi>)
        n16 = property class="Bool (strict)"(reference=w38, error in=w35, "Value"=FALSE) -> (error out=w37:errorcluster)  [unwired: 1 out]
        n17 = Merge Errors(w32, w37) -> (w36:errorcluster)
      }
      frame "Set Interface" {
        n18 = call "BISS Set Interface.vi"("Error In"=w45, "pcInterfaceOption"="pcInterfaceOption", "ulInterface"="BISS_InterfaceEnum", "ulBISSHandle"=w44) -> ("Error Out"=w43:errorcluster)  [unwired: 5 in, 2 out]
        n19 = call <vilib>:"Clear Errors.vi"("error in (no error)"=w43) -> ("error out"=w48:errorcluster)  [unwired: 5 in, 1 out]
        n20 = control-ref of="Set Interface"() -> (w49:refnum<vi>)
        n21 = property class="Bool (strict)"(reference=w49, error in=w48, "Value"=FALSE) -> (error out=w46:errorcluster)  [unwired: 1 out]
        n22 = Merge Errors(w43, w46) -> (w47:errorcluster)
      }
      frame "Get Interface" {
        n23 = call "BISS Get Interface.vi"("Error In"=w55, "ulBISSHandle"=w53) -> ("Error Out"=w54:errorcluster, "pulInterface"=→"BISS_InterfaceEnum":u32)  [unwired: 6 in, 2 out]
        n24 = call <vilib>:"Clear Errors.vi"("error in (no error)"=w54) -> ("error out"=w56:errorcluster)  [unwired: 5 in, 1 out]
        n25 = control-ref of="Get Interface"() -> (w59:refnum<vi>)
        n26 = property class="Bool (strict)"(reference=w59, error in=w56, "Value"=FALSE) -> (error out=w58:errorcluster)  [unwired: 1 out]
        n27 = Merge Errors(w54, w58) -> (w57:errorcluster)
      }
      frame "Get Interface Info" {
        n28 = call "BiSS Get Interface Info.vi"("Error In"=w66, "ulIndex"="BISS_InterfaceInfoEnum", "ulBISSHandle"=w64) -> ("Error Out"=w65:errorcluster, "pcInterfaceInfo"=→"pcInterfaceInfo":string)  [unwired: 5 in, 2 out]
        n29 = call <vilib>:"Clear Errors.vi"("error in (no error)"=w65) -> ("error out"=w67:errorcluster)  [unwired: 5 in, 1 out]
        n30 = control-ref of="Get Interface Info"() -> (w70:refnum<vi>)
        n31 = property class="Bool (strict)"(reference=w70, error in=w67, "Value"=FALSE) -> (error out=w69:errorcluster)  [unwired: 1 out]
        n32 = Merge Errors(w65, w69) -> (w68:errorcluster)
      }
      frame "Auto Detection" {
        n33 = Path To String(path="pcFilename") -> (string=w76:string)
        n34 = call "BISS Auto Detection.vi"("Error In"=w79, "ulWriteMasterParams"="ulWriteMasterParams", "pcFilename"=w76, "ulBISSHandle"=w78) -> ("Error Out"=w73:errorcluster, "pulSlaveCount"=→"pulSlaveCount":u32)  [unwired: 4 in, 2 out]
        n35 = call <vilib>:"Clear Errors.vi"("error in (no error)"=w73) -> ("error out"=w80:errorcluster)  [unwired: 5 in, 1 out]
        n36 = control-ref of="Auto Detection"() -> (w83:refnum<vi>)
        n37 = property class="Bool (strict)"(reference=w83, error in=w80, "Value"=FALSE) -> (error out=w81:errorcluster)  [unwired: 1 out]
        n38 = Merge Errors(w73, w81) -> (w82:errorcluster)
      }
      frame "Set Com Param" {
        n39 = call "BISS Set Com Param.vi"("Error In"=w90, "ulValue"="ulValue", "ulParam"="BISS_ComParamEnum", "ulBISSHandle"=w89) -> ("Error Out"=w88:errorcluster)  [unwired: 5 in, 2 out]
        n40 = call <vilib>:"Clear Errors.vi"("error in (no error)"=w88) -> ("error out"=w91:errorcluster)  [unwired: 5 in, 1 out]
        n41 = control-ref of="Set Com Param"() -> (w94:refnum<vi>)
        n42 = property class="Bool (strict)"(reference=w94, error in=w91, "Value"=FALSE) -> (error out=w92:errorcluster)  [unwired: 1 out]
        n43 = Merge Errors(w88, w92) -> (w93:errorcluster)
      }
      frame "Get Com Param" {
        n44 = call "BISS Get Com Param.vi"("Error In"=w100, "ulParam"="BISS_ComParamEnum", "ulBISSHandle"=w101) -> ("Error Out"=w99:errorcluster, "pulValue"=→"pulValue":u32)  [unwired: 5 in, 2 out]
        n45 = call <vilib>:"Clear Errors.vi"("error in (no error)"=w99) -> ("error out"=w102:errorcluster)  [unwired: 5 in, 1 out]
        n46 = control-ref of="Get Com Param"() -> (w105:refnum<vi>)
        n47 = property class="Bool (strict)"(reference=w105, error in=w102, "Value"=FALSE) -> (error out=w103:errorcluster)  [unwired: 1 out]
        n48 = Merge Errors(w99, w103) -> (w104:errorcluster)
      }
      frame "Set Frame Param" {
        n49 = call "BISS Set Frame Param.vi"("ulValue"="ulValue", "Error In"=w113, "ulParam"="BISS_FrameParamEnum", "ulDataChannel"="ulDataChannel", "ulBISSHandle"=w112) -> ("Error Out"=w108:errorcluster)  [unwired: 4 in, 2 out]
        n50 = call <vilib>:"Clear Errors.vi"("error in (no error)"=w108) -> ("error out"=w114:errorcluster)  [unwired: 5 in, 1 out]
        n51 = control-ref of="Set Frame Param"() -> (w117:refnum<vi>)
        n52 = property class="Bool (strict)"(reference=w117, error in=w114, "Value"=FALSE) -> (error out=w115:errorcluster)  [unwired: 1 out]
        n53 = Merge Errors(w108, w115) -> (w116:errorcluster)
      }
      frame "Get Frame Param" {
        n54 = call "BISS Get Frame Param.vi"("Error In"=w125, "ulParam"="BISS_FrameParamEnum", "ulDataChannel"="ulDataChannel", "ulBISSHandle"=w124) -> ("Error Out"=w120:errorcluster, "pulValue"=→"pulValue":u32)  [unwired: 4 in, 2 out]
        n55 = call <vilib>:"Clear Errors.vi"("error in (no error)"=w120) -> ("error out"=w126:errorcluster)  [unwired: 5 in, 1 out]
        n56 = control-ref of="Get Frame Param"() -> (w129:refnum<vi>)
        n57 = property class="Bool (strict)"(reference=w129, error in=w126, "Value"=FALSE) -> (error out=w127:errorcluster)  [unwired: 1 out]
        n58 = Merge Errors(w120, w127) -> (w128:errorcluster)
      }
      frame "Write Master Params" {
        n59 = call "BISS Write Master Params.vi"("Error In"=w135, "ulBISSHandle"=w133) -> ("Error Out"=w134:errorcluster)  [unwired: 7 in, 2 out]
        n60 = call <vilib>:"Clear Errors.vi"("error in (no error)"=w134) -> ("error out"=w136:errorcluster)  [unwired: 5 in, 1 out]
        n61 = control-ref of="Write Master Params"() -> (w132:refnum<vi>)
        n62 = property class="Bool (strict)"(reference=w132, error in=w136, "Value"=FALSE) -> (error out=w137:errorcluster)  [unwired: 1 out]
        n63 = Merge Errors(w134, w137) -> (w138:errorcluster)
      }
      frame "Set FTDI Freq" {
        n64 = call "BISS Set Ftdi Freq.vi"("Error In"=w146, "ulFreqL"="ulFreqL", "ulFreqH"="ulFreqH", "ulBISSHandle"=w144) -> ("Error Out"=w145:errorcluster)  [unwired: 6 in, 1 out]
        n65 = call <vilib>:"Clear Errors.vi"("error in (no error)"=w145) -> ("error out"=w150:errorcluster)  [unwired: 5 in, 1 out]
        n66 = control-ref of="Set FTDI Freq"() -> (w141:refnum<vi>)
        n67 = property class="Bool (strict)"(reference=w141, error in=w150, "Value"=FALSE) -> (error out=w148:errorcluster)  [unwired: 1 out]
        n68 = Merge Errors(w145, w148) -> (w147:errorcluster)
      }
      frame "Init BiSS Comm" {
        n69 = call "BISS Init Biss Comm.vi"("Error In"=w156, "ulBiSSHandle"=w155) -> ("Error Out"=w154:errorcluster)  [unwired: 7 in, 2 out]
        n70 = call <vilib>:"Clear Errors.vi"("error in (no error)"=w154) -> ("error out"=w157:errorcluster)  [unwired: 5 in, 1 out]
        n71 = control-ref of="Init BiSS Comm"() -> (w158:refnum<vi>)
        n72 = property class="Bool (strict)"(reference=w158, error in=w157, "Value"=FALSE) -> (error out=w153:errorcluster)  [unwired: 1 out]
        n73 = Merge Errors(w154, w153) -> (w152:errorcluster)
      }
      frame "Write Slave Register" {
        n74 = call "BISS Write Slave Register.vi"("pulRegisterContent"="pulRegisterContent", "pulNumberOfBytes"="pulNumberOfBytes", "ulRegisterAddress"="ulRegisterAddress", "Error In"=w169, "ulSlaveId"="ulSlaveId", "ulProtocol"="ulProtocol", "ulBISSHandle"=w167) -> ("Error Out"=w168:errorcluster, "pulNumberOfBytes out"=w161:u32)  [unwired: 1 in, 2 out]
        n75 = property on="pulNumberOfBytes" class="DigNum (strict)"("Value"=w161) -> ()  [unwired: 2 in, 2 out]
        n76 = call <vilib>:"Clear Errors.vi"("error in (no error)"=w168) -> ("error out"=w172:errorcluster)  [unwired: 5 in, 1 out]
        n77 = control-ref of="Write Slave Register"() -> (w173:refnum<vi>)
        n78 = property class="Bool (strict)"(reference=w173, error in=w172, "Value"=FALSE) -> (error out=w171:errorcluster)  [unwired: 1 out]
        n79 = Merge Errors(w168, w171) -> (w170:errorcluster)
      }
      frame "Read Slave Register" {
        n80 = call "BISS Read Slave Register.vi"("pulNumberOfBytes"="pulNumberOfBytes", "ulRegisterAddress"="ulRegisterAddress", "Error In"=w184, "ulSlaveId"="ulSlaveId", "ulProtocol"="ulProtocol", "ulBISSHandle"=w185) -> ("Error Out"=w183:errorcluster, "pulRegisterContent"=→"pulRegisterContent":u32[], "pulNumberOfBytes"=w177:u32)  [unwired: 1 in, 2 out]
        n81 = property on="pulNumberOfBytes" class="DigNum (strict)"("Value"=w177) -> ()  [unwired: 2 in, 2 out]
        n82 = call <vilib>:"Clear Errors.vi"("error in (no error)"=w183) -> ("error out"=w187:errorcluster)  [unwired: 5 in, 1 out]
        n83 = control-ref of="Read Slave Register"() -> (w188:refnum<vi>)
        n84 = property class="Bool (strict)"(reference=w188, error in=w187, "Value"=FALSE) -> (error out=w186:errorcluster)  [unwired: 1 out]
        n85 = Merge Errors(w183, w186) -> (w182:errorcluster)
      }
      frame "Read SCD" {
        n86 = call "BISS Read SCD.vi"("Error In"=w198, "ulStartControlFrame"="ulStartControlFrame", "ulBISSHandle"=w196) -> ("Error Out"=w197:errorcluster, "pulDataScdL"=→"pulDataScdL":u32[], "pulDataScdH"=→"pulDataScdH":u32[], "pulScdValid"=→"pulScdValid":u32, "pulControlFrameEnd"=→"pulControlFrameEnd":u32)  [unwired: 3 in, 1 out]
        n87 = call <vilib>:"Clear Errors.vi"("error in (no error)"=w197) -> ("error out"=w201:errorcluster)  [unwired: 5 in, 1 out]
        n88 = control-ref of="Read SCD"() -> (w202:refnum<vi>)
        n89 = property class="Bool (strict)"(reference=w202, error in=w201, "Value"=FALSE) -> (error out=w199:errorcluster)  [unwired: 1 out]
        n90 = Merge Errors(w197, w199) -> (w200:errorcluster)
      }
      frame "Send Command" {
        n91 = call "BISS Send Command.vi"("Error In"=w208, "ulCmd"="ulCmd", "ulIds"="ulIds", "ulBISSHandle"=w209) -> ("Error Out"=w207:errorcluster)  [unwired: 5 in, 2 out]
        n92 = call <vilib>:"Clear Errors.vi"("error in (no error)"=w207) -> ("error out"=w212:errorcluster)  [unwired: 5 in, 1 out]
        n93 = control-ref of="Send Command"() -> (w213:refnum<vi>)
        n94 = property class="Bool (strict)"(reference=w213, error in=w212, "Value"=FALSE) -> (error out=w211:errorcluster)  [unwired: 1 out]
        n95 = Merge Errors(w207, w211) -> (w210:errorcluster)
      }
      frame "Set Slave Label" {
        n96 = call "BISS Set Slave Label.vi"("pcManufacturerLabel"="pcManufacturerLabel", "pcCompleteLabel"="pcCompleteLabel", "Error In"=w222, "pcSlaveLabel"="pcSlaveLabel", "ulSlave"="ulSlave", "ulBISSHandle"=w221) -> ("Error Out"=w220:errorcluster)  [unwired: 4 in, 1 out]
        n97 = call <vilib>:"Clear Errors.vi"("error in (no error)"=w220) -> ("error out"=w225:errorcluster)  [unwired: 5 in, 1 out]
        n98 = control-ref of="Set Slave Label"() -> (w226:refnum<vi>)
        n99 = property class="Bool (strict)"(reference=w226, error in=w225, "Value"=FALSE) -> (error out=w223:errorcluster)  [unwired: 1 out]
        n100 = Merge Errors(w220, w223) -> (w224:errorcluster)
      }
      frame "Get Slave Label" {
        n101 = call "BISS Get Slave Label.vi"("Error In"=w235, "ulSlave"="ulSlave 2", "ulBISSHandle"=w236) -> ("Error Out"=w234:errorcluster, "pcSlaveLabel"=→"pcSlaveLabel 2":string, "pcManufacturerLabel"=→"pcManufacturerLabel 2":string, "pcCompleteLabel"=→"pcCompleteLabel 2":string)  [unwired: 3 in, 2 out]
        n102 = call <vilib>:"Clear Errors.vi"("error in (no error)"=w234) -> ("error out"=w237:errorcluster)  [unwired: 5 in, 1 out]
        n103 = control-ref of="Get Slave Label"() -> (w233:refnum<vi>)
        n104 = property class="Bool (strict)"(reference=w233, error in=w237, "Value"=FALSE) -> (error out=w238:errorcluster)  [unwired: 1 out]
        n105 = Merge Errors(w234, w238) -> (w239:errorcluster)
      }
      frame "Set SCD Content Labels" {
        n106 = call "BISS Set SCD Content Labels.vi"("pcScdContentUnit"="pcScdContentUnit", "pcScdContentLabel"="pcScdContentLabel", "Error In"=w248, "ulContentIndex"="ulContentIndex", "ulDataChannel"="ulDataChannel", "ulBISSHandle"=w246) -> ("Error Out"=w247:errorcluster)  [unwired: 3 in, 2 out]
        n107 = call <vilib>:"Clear Errors.vi"("error in (no error)"=w247) -> ("error out"=w251:errorcluster)  [unwired: 5 in, 1 out]
        n108 = control-ref of="Set SCD Content Labels"() -> (w252:refnum<vi>)
        n109 = property class="Bool (strict)"(reference=w252, error in=w251, "Value"=FALSE) -> (error out=w249:errorcluster)  [unwired: 1 out]
        n110 = Merge Errors(w247, w249) -> (w250:errorcluster)
      }
      frame "Get SCD Content Labels" {
        n111 = call "BISS Get SCD Content Labels.vi"("Error In"=w261, "ulContentIndex"="ulContentIndex", "ulDataChannel"="ulDataChannel", "ulBISSHandle"=w259) -> ("Error Out"=w260:errorcluster, "pcSCDContentUnit"=→"pcSCDContentUnit":string, "pcSCDContentLabel"=→"pcSCDContentLabel":string)  [unwired: 3 in, 2 out]
        n112 = call <vilib>:"Clear Errors.vi"("error in (no error)"=w260) -> ("error out"=w264:errorcluster)  [unwired: 5 in, 1 out]
        n113 = control-ref of="Get SCD Content Labels"() -> (w265:refnum<vi>)
        n114 = property class="Bool (strict)"(reference=w265, error in=w264, "Value"=FALSE) -> (error out=w262:errorcluster)  [unwired: 1 out]
        n115 = Merge Errors(w260, w262) -> (w263:errorcluster)
      }
      frame "Get SCD Content" {
        n116 = call "BISS Get SCD Content.vi"("Error In"=w272, "ulDataChannel"="ulDataChannel", "ulBISSHandle"=w270) -> ("Error Out"=w271:errorcluster, "pulScdContentValues"=→"pulScdContentValues":u32[])  [unwired: 5 in, 2 out]
        n117 = call <vilib>:"Clear Errors.vi"("error in (no error)"=w271) -> ("error out"=w275:errorcluster)  [unwired: 5 in, 1 out]
        n118 = control-ref of="Get SCD Content"() -> (w276:refnum<vi>)
        n119 = property class="Bool (strict)"(reference=w276, error in=w275, "Value"=FALSE) -> (error out=w273:errorcluster)  [unwired: 1 out]
        n120 = Merge Errors(w271, w273) -> (w274:errorcluster)
      }
      frame "Get SCD Content Ex" {
        n121 = call "BISS Get SCD Content Ex.vi"("Error In"=w283, "ulDataChannel"="ulDataChannel", "ulBISSHandle"=w281) -> ("Error Out"=w282:errorcluster, "pulScdContentValues"=→"pulScdContentValues":u64[])  [unwired: 6 in, 1 out]
        n122 = call <vilib>:"Clear Errors.vi"("error in (no error)"=w282) -> ("error out"=w286:errorcluster)  [unwired: 5 in, 1 out]
        n123 = control-ref of="Get SCD Content Ex"() -> (w287:refnum<vi>)
        n124 = property class="Bool (strict)"(reference=w287, error in=w286, "Value"=FALSE) -> (error out=w284:errorcluster)  [unwired: 1 out]
        n125 = Merge Errors(w282, w284) -> (w285:errorcluster)
      }
      frame "Set SCD Content Params" {
        n126 = call "BISS Set SCD Content Params.vi"("pScdContentItems"="pScdContentItems", "Error In"=w295, "ulContentIndex"="ulContentIndex", "ulDataChannel"="ulDataChannel", "ulBISSHandle"=w293) -> ("Error Out"=w294:errorcluster)  [unwired: 4 in, 2 out]
        n127 = call <vilib>:"Clear Errors.vi"("error in (no error)"=w294) -> ("error out"=w298:errorcluster)  [unwired: 5 in, 1 out]
        n128 = control-ref of="Set SCD Content Params"() -> (w299:refnum<vi>)
        n129 = property class="Bool (strict)"(reference=w299, error in=w298, "Value"=FALSE) -> (error out=w296:errorcluster)  [unwired: 1 out]
        n130 = Merge Errors(w294, w296) -> (w297:errorcluster)
      }
      frame "Get SCD Content Params" {
        n131 = call "BISS Get SCD Content Params.vi"("Error In"=w307, "ulContentIndex"="ulContentIndex", "ulDataChannel"="ulDataChannel", "ulBISSHandle"=w305) -> ("Error Out"=w306:errorcluster, "pScdContentItems out"=→"pScdContentItems":T7)  [unwired: 4 in, 2 out]
        n132 = call <vilib>:"Clear Errors.vi"("error in (no error)"=w306) -> ("error out"=w310:errorcluster)  [unwired: 5 in, 1 out]
        n133 = control-ref of="Get SCD Content Params"() -> (w311:refnum<vi>)
        n134 = property class="Bool (strict)"(reference=w311, error in=w310, "Value"=FALSE) -> (error out=w308:errorcluster)  [unwired: 1 out]
        n135 = Merge Errors(w306, w308) -> (w309:errorcluster)
      }
      frame "Read SCD Frames" {
        n136 = Tick Count (ms)() -> (millisecond timer value=w314:u32)
        n137 = while {
          tunnel: w316 -> [w343]
          shift-right: [w342] -> w315
          shift-left: w317 -> [w344]
          tunnel: [w321] -> _
          tunnel: w314 -> [w320]
          stop <- "stop" stop-if-true
          n138 = Tick Count (ms)() -> (millisecond timer value=w321:u32)
          n139 = call "BISS Read SCD Frames.vi"("Error In"=w344, "ulCycleCnt"="ulCycleCnt", "ulBISSHandle"=w343) -> ("Error Out"=w334:errorcluster, "pulDataScdL"=w339:u32[], "pulDataScdH"=→"pulDataScdH":u32[], "pulTimestamp"=→"pulTimestamp":u32[], "pulStatus"=→"pulStatus":u32[])  [unwired: 3 in, 1 out]
          n140 = Subtract(x=w321, y=w320) -> (x-y=→"Loop Time [ms]":u32)
          n141 = Wait Until Next ms Multiple(millisecond multiple="Update Time [ms]") -> ()  [unwired: 1 out]
          n142 = Logical Shift(y=-2, x=w339) -> (x << y=w340:u32[])
          n143 = To Single Precision Float(number=w340) -> (single precision float=w341:sgl[])
          n144 = Get Date/Time In Seconds() -> (seconds since 1Jan1904=w326:timestamp)
          n145 = call <vilib>:"Clear Errors.vi"("error in (no error)"=w334) -> ("error out"=w332:errorcluster)  [unwired: 5 in, 1 out]
          n146 = Divide(x=w341, y=1000000) -> (x/y=w319:sgl[])
          "pulDataScdL" <- w319
          n147 = Bundle By Name("t0"=w326, "Y"=w319, "dt"=1) -> (→"Displacement vs Time":waveform(sgl))  [unwired: 1 in]
          n148 = control-ref of="Read SCD Frames"() -> (w331:refnum<vi>)
          n149 = property class="Bool (strict)"(reference=w331, error in=w332, "Value"=FALSE) -> (error out=w333:errorcluster)  [unwired: 1 out]
          n150 = Merge Errors(w334, w333) -> (w342:errorcluster)
        }
      }
      frame "Get SCD Frame" {
        n151 = call "BiSS Get SCD Frame.vi"("Error In"=w351, "ulFrameIndex"="ulFrameIndex", "ulBISSHandle"=w352) -> ("Error Out"=w350:errorcluster, "pulDataScdL"=→"pulDataScdL":u32[], "pulDataScdH"=→"pulDataScdH":u32[], "pulStatus"=→"pulStatus":u32, "pulTimestamp"=→"pulTimestamp":u32)  [unwired: 2 in, 2 out]
        n152 = call <vilib>:"Clear Errors.vi"("error in (no error)"=w350) -> ("error out"=w355:errorcluster)  [unwired: 5 in, 1 out]
        n153 = control-ref of="Get SCD Frame"() -> (w356:refnum<vi>)
        n154 = property class="Bool (strict)"(reference=w356, error in=w355, "Value"=FALSE) -> (error out=w353:errorcluster)  [unwired: 1 out]
        n155 = Merge Errors(w350, w353) -> (w354:errorcluster)
      }
      frame "Get SCD Frame Ex" {
        n156 = call "BISS Get SCD Frame Ex.vi"("ulCycleCount"="ulCycleCount", "Error In"=w367, "ulDataChannel"="ulDataChannel", "ulBISSHandle"=w365) -> ("Error Out"=w366:errorcluster, "pulDataScdL"=→"pulDataScdL":u32[], "pulDataScdH"=→"pulDataScdH":u32[], "pulTimestamp"=→"pulTimestamp":u32[], "pulStatus"=→"pulStatus":u32[])  [unwired: 2 in, 1 out]
        n157 = call <vilib>:"Clear Errors.vi"("error in (no error)"=w366) -> ("error out"=w370:errorcluster)  [unwired: 5 in, 1 out]
        n158 = control-ref of="Get SCD Frame Ex"() -> (w371:refnum<vi>)
        n159 = property class="Bool (strict)"(reference=w371, error in=w370, "Value"=FALSE) -> (error out=w368:errorcluster)  [unwired: 1 out]
        n160 = Merge Errors(w366, w368) -> (w369:errorcluster)
      }
      frame "Get SCD Frame Content" {
        n161 = call "BISS Get SCD Frame Content.vi"("ulCycleCount"="ulCycleCount", "Error In"=w380, "ulContentIndex"="ulContentIndex", "ulDataChannel"="ulDataChannel", "ulBISSHandle"=w378) -> ("Error Out"=w379:errorcluster, "pulValues"=→"pulValues":u32[])  [unwired: 3 in, 2 out]
        n162 = call <vilib>:"Clear Errors.vi"("error in (no error)"=w379) -> ("error out"=w383:errorcluster)  [unwired: 5 in, 1 out]
        n163 = control-ref of="Get SCD Frame Content"() -> (w384:refnum<vi>)
        n164 = property class="Bool (strict)"(reference=w384, error in=w383, "Value"=FALSE) -> (error out=w381:errorcluster)  [unwired: 1 out]
        n165 = Merge Errors(w379, w381) -> (w382:errorcluster)
      }
      frame "Get SCD Frame Content Ex" {
        n166 = call "BISS Get SCD Frame Content Ex.vi"("ulCycleCount"="ulCycleCount", "Error In"=w398, "ulContentIndex"="ulContentIndex", "ulDataChannel"="ulDataChannel", "ulBISSHandle"=w397) -> ("Error Out"=w389:errorcluster, "pulValues"=→"pulValues":u64[])  [unwired: 4 in, 1 out]
        n167 = call <vilib>:"Clear Errors.vi"("error in (no error)"=w389) -> ("error out"=w392:errorcluster)  [unwired: 5 in, 1 out]
        n168 = control-ref of="Get SCD Frame Content Ex"() -> (w387:refnum<vi>)
        n169 = property class="Bool (strict)"(reference=w387, error in=w392, "Value"=FALSE) -> (error out=w391:errorcluster)  [unwired: 1 out]
        n170 = Merge Errors(w389, w391) -> (w388:errorcluster)
      }
      frame "Set EDS Param" {
        n171 = call "BISS Set EDS Param.vi"("Error In"=w404, "ulValue"="ulValue", "ulParam"="BISS_EdsParamEnum", "ulBISSHandle"=w402) -> ("Error Out"=w403:errorcluster)  [unwired: 6 in, 1 out]
        n172 = call <vilib>:"Clear Errors.vi"("error in (no error)"=w403) -> ("error out"=w407:errorcluster)  [unwired: 5 in, 1 out]
        n173 = control-ref of="Set EDS Param"() -> (w408:refnum<vi>)
        n174 = property class="Bool (strict)"(reference=w408, error in=w407, "Value"=FALSE) -> (error out=w406:errorcluster)  [unwired: 1 out]
        n175 = Merge Errors(w403, w406) -> (w405:errorcluster)
      }
      frame "Get EDS Param" {
        n176 = call "BISS Get EDS Param.vi"("Error In"=w415, "ulParam"="BISS_EdsParamEnum", "ulBISSHandle"=w413) -> ("Error Out"=w414:errorcluster, "pulValue"=→"pulValue":u32)  [unwired: 6 in, 1 out]
        n177 = call <vilib>:"Clear Errors.vi"("error in (no error)"=w414) -> ("error out"=w418:errorcluster)  [unwired: 5 in, 1 out]
        n178 = control-ref of="Get EDS Param"() -> (w419:refnum<vi>)
        n179 = property class="Bool (strict)"(reference=w419, error in=w418, "Value"=FALSE) -> (error out=w417:errorcluster)  [unwired: 1 out]
        n180 = Merge Errors(w414, w417) -> (w416:errorcluster)
      }
      frame "Set EDS Register" {
        n181 = call "BISS Set EDS Register.vi"("Error In"=w425, "ulValue"="ulValue", "ulAdr"="ulAdr", "ulBISSHandle"=w426) -> ("Error Out"=w424:errorcluster)  [unwired: 6 in, 1 out]
        n182 = call <vilib>:"Clear Errors.vi"("error in (no error)"=w424) -> ("error out"=w429:errorcluster)  [unwired: 5 in, 1 out]
        n183 = control-ref of="Set EDS Register"() -> (w430:refnum<vi>)
        n184 = property class="Bool (strict)"(reference=w430, error in=w429, "Value"=FALSE) -> (error out=w428:errorcluster)  [unwired: 1 out]
        n185 = Merge Errors(w424, w428) -> (w427:errorcluster)
      }
      frame "Get EDS Register" {
        n186 = call "BISS Get EDS Register.vi"("Error In"=w436, "ulAdr"="ulAdr", "ulBISSHandle"=w437) -> ("Error Out"=w435:errorcluster, "pulValue"=→"pulValue":u32)  [unwired: 6 in, 1 out]
        n187 = call <vilib>:"Clear Errors.vi"("error in (no error)"=w435) -> ("error out"=w440:errorcluster)  [unwired: 5 in, 1 out]
        n188 = control-ref of="Get EDS Register"() -> (w441:refnum<vi>)
        n189 = property class="Bool (strict)"(reference=w441, error in=w440, "Value"=FALSE) -> (error out=w439:errorcluster)  [unwired: 1 out]
        n190 = Merge Errors(w435, w439) -> (w438:errorcluster)
      }
      frame "Read EDS Params" {
        n191 = call "BISS Read EDS Params.vi"("Error In"=w447, "ulSlaveId"="ulSlaveId", "ulBISSHandle"=w445) -> ("Error Out"=w446:errorcluster)  [unwired: 7 in, 1 out]
        n192 = call <vilib>:"Clear Errors.vi"("error in (no error)"=w446) -> ("error out"=w450:errorcluster)  [unwired: 5 in, 1 out]
        n193 = control-ref of="Read EDS Params"() -> (w451:refnum<vi>)
        n194 = property class="Bool (strict)"(reference=w451, error in=w450, "Value"=FALSE) -> (error out=w449:errorcluster)  [unwired: 1 out]
        n195 = Merge Errors(w446, w449) -> (w448:errorcluster)
      }
      frame "Write EDS Params" {
        n196 = call "BISS Write EDS Params.vi"("Error In"=w457, "ulSlaveId"="ulSlaveId", "ulBISSHandle"=w455) -> ("Error Out"=w456:errorcluster)  [unwired: 7 in, 1 out]
        n197 = call <vilib>:"Clear Errors.vi"("error in (no error)"=w456) -> ("error out"=w460:errorcluster)  [unwired: 5 in, 1 out]
        n198 = control-ref of="Write EDS Params"() -> (w461:refnum<vi>)
        n199 = property class="Bool (strict)"(reference=w461, error in=w460, "Value"=FALSE) -> (error out=w459:errorcluster)  [unwired: 1 out]
        n200 = Merge Errors(w456, w459) -> (w458:errorcluster)
      }
      frame "Get DLL Version" {
        n201 = call "BISS Get DLL Version.vi"("Error In"=w466) -> ("Error Out"=w465:errorcluster, "pulDllVersion"=→"pulDllVersion":u32[])  [unwired: 7 in, 2 out]
        n202 = call <vilib>:"Clear Errors.vi"("error in (no error)"=w465) -> ("error out"=w470:errorcluster)  [unwired: 5 in, 1 out]
        n203 = control-ref of="Get DLL Version"() -> (w471:refnum<vi>)
        n204 = property class="Bool (strict)"(reference=w471, error in=w470, "Value"=FALSE) -> (error out=w469:errorcluster)  [unwired: 1 out]
        n205 = Merge Errors(w465, w469) -> (w468:errorcluster)
      }
      frame "Calculate CRC" {
        n206 = call "BISS Calculate CRC.vi"("ulByteCount"="ulByteCount", "Error In"=w480, "pulData"="pulData", "ulCrcPoly"="ulCrcPoly", "ulBISSHandle"=w478) -> ("Error Out"=w479:errorcluster, "pulCheckSum"=→"pulCheckSum":u32)  [unwired: 4 in, 1 out]
        n207 = call <vilib>:"Clear Errors.vi"("error in (no error)"=w479) -> ("error out"=w483:errorcluster)  [unwired: 5 in, 1 out]
        n208 = control-ref of="Calculate CRC"() -> (w484:refnum<vi>)
        n209 = property class="Bool (strict)"(reference=w484, error in=w483, "Value"=FALSE) -> (error out=w482:errorcluster)  [unwired: 1 out]
        n210 = Merge Errors(w479, w482) -> (w481:errorcluster)
      }
      frame "Calculate CRC Ex" {
        n211 = call "BISS Calculate CRC Ex.vi"("ulCRCStartValue"="ulCRCStartValue", "ulByteCount"="ulByteCount", "Error In"=w494, "pulData"="pulData", "ulCrcPoly"="ulCrcPoly", "ulBISSHandle"=w492) -> ("Error Out"=w493:errorcluster, "pulCheckSum"=→"pulCheckSum":u32)  [unwired: 3 in, 1 out]
        n212 = call <vilib>:"Clear Errors.vi"("error in (no error)"=w493) -> ("error out"=w497:errorcluster)  [unwired: 5 in, 1 out]
        n213 = control-ref of="Calculate CRC Ex"() -> (w498:refnum<vi>)
        n214 = property class="Bool (strict)"(reference=w498, error in=w497, "Value"=FALSE) -> (error out=w496:errorcluster)  [unwired: 1 out]
        n215 = Merge Errors(w493, w496) -> (w495:errorcluster)
      }
      frame "Save DLL Config" {
        n216 = Path To String(path="pcFilename") -> (string=w503:string)
        n217 = call "BISS Save DLL Config.vi"("Error In"=w505, "pcCfgFilename"=w503, "ulBISSHandle"=w506) -> ("Error Out"=w504:errorcluster)  [unwired: 7 in, 1 out]
        n218 = call <vilib>:"Clear Errors.vi"("error in (no error)"=w504) -> ("error out"=w509:errorcluster)  [unwired: 5 in, 1 out]
        n219 = control-ref of="Save DLL Config"() -> (w501:refnum<vi>)
        n220 = property class="Bool (strict)"(reference=w501, error in=w509, "Value"=FALSE) -> (error out=w508:errorcluster)  [unwired: 1 out]
        n221 = Merge Errors(w504, w508) -> (w507:errorcluster)
      }
      frame "Load DLL Config" {
        n222 = Path To String(path="pcFilename 2") -> (string=w514:string)
        n223 = call "BISS Load DLL Config.vi"("Error In"=w516, "pcCfgFilename"=w514, "ulBISSHandle"=w517) -> ("Error Out"=w515:errorcluster)  [unwired: 7 in, 1 out]
        n224 = call <vilib>:"Clear Errors.vi"("error in (no error)"=w515) -> ("error out"=w520:errorcluster)  [unwired: 5 in, 1 out]
        n225 = control-ref of="Load DLL Config"() -> (w513:refnum<vi>)
        n226 = property class="Bool (strict)"(reference=w513, error in=w520, "Value"=FALSE) -> (error out=w519:errorcluster)  [unwired: 1 out]
        n227 = Merge Errors(w515, w519) -> (w518:errorcluster)
      }
      frame "Get Last Error" {
        n228 = call "BISS Get Last Error.vi"("Error In"=w528, "ulBISSHandle"=w526) -> ("Error Out"=w527:errorcluster, "pulErrorType"=→"BISS_ErrorTypeEnum":u32, "pulLastError"=→"pulLastError":u32, "pcErrorText"=→"pcErrorText":string)  [unwired: 5 in, 1 out]
        n229 = call <vilib>:"Clear Errors.vi"("error in (no error)"=w527) -> ("error out"=w531:errorcluster)  [unwired: 5 in, 1 out]
        n230 = control-ref of="Get Last Error"() -> (w532:refnum<vi>)
        n231 = property class="Bool (strict)"(reference=w532, error in=w531, "Value"=FALSE) -> (error out=w530:errorcluster)  [unwired: 1 out]
        n232 = Merge Errors(w527, w530) -> (w529:errorcluster)
      }
      frame "Get MB3U Pins" {
        n233 = call "BISS Get MB3U Pins.vi"("Error In"=w539, "ulBISSHandle"=w537) -> ("Error Out"=w538:errorcluster, "pulValue"=→"pulValue":u32, "pulDir"=→"pulDir":u32)  [unwired: 6 in, 1 out]
        n234 = call <vilib>:"Clear Errors.vi"("error in (no error)"=w538) -> ("error out"=w542:errorcluster)  [unwired: 5 in, 1 out]
        n235 = control-ref of="Get MB3U Pins"() -> (w543:refnum<vi>)
        n236 = property class="Bool (strict)"(reference=w543, error in=w542, "Value"=FALSE) -> (error out=w541:errorcluster)  [unwired: 1 out]
        n237 = Merge Errors(w538, w541) -> (w540:errorcluster)
      }
      frame "Set MB3U Pins" {
        n238 = call "BISS Set MB3U Pins.vi"("Error In"=w550, "ulValue"="ulValue", "ulDir"="ulDir", "ulBISSHandle"=w548) -> ("Error Out"=w549:errorcluster)  [unwired: 6 in, 1 out]
        n239 = call <vilib>:"Clear Errors.vi"("error in (no error)"=w549) -> ("error out"=w553:errorcluster)  [unwired: 5 in, 1 out]
        n240 = control-ref of="Set MB3U Pins"() -> (w554:refnum<vi>)
        n241 = property class="Bool (strict)"(reference=w554, error in=w553, "Value"=FALSE) -> (error out=w552:errorcluster)  [unwired: 1 out]
        n242 = Merge Errors(w549, w552) -> (w551:errorcluster)
      }
      frame "Write Master Register" {
        n243 = call "BISS Write Master Register.vi"("Error In"=w561, "ulRegisterContent"="ulRegisterContent", "ulRegisterAddress"="ulRegisterAddress", "ulBISSHandle"=w559) -> ("Error Out"=w560:errorcluster)  [unwired: 5 in, 2 out]
        n244 = call <vilib>:"Clear Errors.vi"("error in (no error)"=w560) -> ("error out"=w564:errorcluster)  [unwired: 5 in, 1 out]
        n245 = control-ref of="Write Master Register"() -> (w565:refnum<vi>)
        n246 = property class="Bool (strict)"(reference=w565, error in=w564, "Value"=FALSE) -> (error out=w563:errorcluster)  [unwired: 1 out]
        n247 = Merge Errors(w560, w563) -> (w562:errorcluster)
      }
      frame "Read Master Register" {
        n248 = call "BISS Read Master Register.vi"("Error In"=w572, "ulRegisterAddress"="ulRegisterAddress", "ulBISSHandle"=w570) -> ("Error Out"=w571:errorcluster, "pulRegisterContent"=→"pulRegisterContent":u32)  [unwired: 5 in, 2 out]
        n249 = call <vilib>:"Clear Errors.vi"("error in (no error)"=w571) -> ("error out"=w575:errorcluster)  [unwired: 5 in, 1 out]
        n250 = control-ref of="Read Master Register"() -> (w576:refnum<vi>)
        n251 = property class="Bool (strict)"(reference=w576, error in=w575, "Value"=FALSE) -> (error out=w574:errorcluster)  [unwired: 1 out]
        n252 = Merge Errors(w571, w574) -> (w573:errorcluster)
      }
      frame "Get Master Register" {
        n253 = call "BISS Get Master Register.vi"("Error In"=w583, "ulRegisterAddress"="ulRegisterAddress", "ulBISSHandle"=w581) -> ("Error Out"=w582:errorcluster, "pulRegisterContent"=→"pulRegisterContent":u32)  [unwired: 5 in, 2 out]
        n254 = call <vilib>:"Clear Errors.vi"("error in (no error)"=w582) -> ("error out"=w586:errorcluster)  [unwired: 5 in, 1 out]
        n255 = control-ref of="Get Master Register"() -> (w587:refnum<vi>)
        n256 = property class="Bool (strict)"(reference=w587, error in=w586, "Value"=FALSE) -> (error out=w585:errorcluster)  [unwired: 1 out]
        n257 = Merge Errors(w582, w585) -> (w584:errorcluster)
      }
      frame "Save Master Config" {
        n258 = Path To String(path="pcFilename") -> (string=w590:string)
        n259 = call "BISS Save Master Config.vi"("Error In"=w594, "pcCfgFilename"=w590, "ulBISSHandle"=w592) -> ("Error Out"=w593:errorcluster)  [unwired: 7 in, 1 out]
        n260 = call <vilib>:"Clear Errors.vi"("error in (no error)"=w593) -> ("error out"=w597:errorcluster)  [unwired: 5 in, 1 out]
        n261 = control-ref of="Save Master Config"() -> (w598:refnum<vi>)
        n262 = property class="Bool (strict)"(reference=w598, error in=w597, "Value"=FALSE) -> (error out=w596:errorcluster)  [unwired: 1 out]
        n263 = Merge Errors(w593, w596) -> (w595:errorcluster)
      }
      frame "Save Register" {
        n264 = Path To String(path="pcFilename") -> (string=w604:string)
        n265 = call "BISS Save Register.vi"("pulData"="pulData", "ulNumberOfBytes"="ulNumberOfBytes", "Error In"=w608, "ulStartAdr"="ulStartAdr", "pcFilename"=w604, "ulBISSHandle"=w606) -> ("Error Out"=w607:errorcluster)  [unwired: 4 in, 1 out]
        n266 = call <vilib>:"Clear Errors.vi"("error in (no error)"=w607) -> ("error out"=w611:errorcluster)  [unwired: 5 in, 1 out]
        n267 = control-ref of="Save Register"() -> (w612:refnum<vi>)
        n268 = property class="Bool (strict)"(reference=w612, error in=w611, "Value"=FALSE) -> (error out=w610:errorcluster)  [unwired: 1 out]
        n269 = Merge Errors(w607, w610) -> (w609:errorcluster)
      }
      frame "Load Register" {
        n270 = Path To String(path="pcFilename") -> (string=w618:string)
        n271 = call "BISS Load Register.vi"("ulNumberOfBytes"="ulNumberOfBytes", "Error In"=w622, "ulStartAdr"="ulStartAdr", "pcFilename"=w618, "ulBISSHandle"=w620) -> ("Error Out"=w621:errorcluster, "pulData"=→"pulData":u32[])  [unwired: 4 in, 1 out]
        n272 = call <vilib>:"Clear Errors.vi"("error in (no error)"=w621) -> ("error out"=w625:errorcluster)  [unwired: 5 in, 1 out]
        n273 = control-ref of="Load Register"() -> (w626:refnum<vi>)
        n274 = property class="Bool (strict)"(reference=w626, error in=w625, "Value"=FALSE) -> (error out=w624:errorcluster)  [unwired: 1 out]
        n275 = Merge Errors(w621, w624) -> (w623:errorcluster)
      }
      frame "Stop Demo" {
        n276 = Release Queue(queue=w635, error in (no error)=w636) -> (error out=w629:errorcluster)  [unwired: 1 in, 2 out]
        n277 = call <vilib>:"Clear Errors.vi"("error in (no error)"=w629) -> ("error out"=w632:errorcluster)  [unwired: 5 in, 1 out]
        n278 = control-ref of="Stop Button"() -> (w631:refnum<vi>)
        n279 = property class="Bool (strict)"(reference=w631, error in=w632, "Value"=FALSE) -> (error out=w633:errorcluster)  [unwired: 1 out]
        n280 = Merge Errors(w629, w633) -> (w634:errorcluster)
      }
    }
    n281 = call <vilib>:"Simple Error Handler.vi"("error in (no error)"=w13) -> ()  [unwired: 4 in, 5 out]
  }
  n282 = while {
    tunnel: w3 -> [w642]
    tunnel: w4 -> [w643]
    tunnel: FALSE -> [w640]
    stop <- w639 stop-if-true
    n283 = event shown="[18] \"Get Slave Label\": Value Change" {
      selector: _ -> [_ _ _ _ _ _ _ _ _ _ _ _ _ _ _ _ _ _ _ _ _ _ _ _ _ _ _ _ _ _ _ _ _ _ _ _ _ _ _ _ _ _ _ _ _ _ _ _ _ _ _]
      dyn-events: _ -> [_ _ _ _ _ _ _ _ _ _ _ _ _ _ _ _ _ _ _ _ _ _ _ _ _ _ _ _ _ _ _ _ _ _ _ _ _ _ _ _ _ _ _ _ _ _ _ _ _ _ _]
      timeout: _ -> [_ _ _ _ _ _ _ _ _ _ _ _ _ _ _ _ _ _ _ _ _ _ _ _ _ _ _ _ _ _ _ _ _ _ _ _ _ _ _ _ _ _ _ _ _ _ _ _ _ _ _]
      tunnel: w642 -> [w648 w653 w658 w663 w668 w672 w678 w683 w687 w693 w698 w703 w708 w713 w718 w723 w728 w733 w738 w743 w748 w753 w756 w761 w766 w771 w776 w781 w786 w792 w796 w801 w806 w811 w816 w821 w826 w831 w836 w841 w846 w851 w856 w861 w866 w871 w876 w881 w886 w891 w897]
      tunnel: [w647 w652 w657 w662 w667 w673 w677 w682 w688 w692 w697 w700 w707 w712 w717 w722 w727 w732 w737 w742 w747 w751 w754 w759 w764 w769 w774 w779 w784 w791 w794 w799 w804 w809 w814 w819 w824 w829 w834 w839 w844 w849 w854 w859 w864 w869 w874 w879 w884 w889 w895] -> w641
      tunnel: w643 -> [w646 w651 w656 w661 w666 w671 w676 w681 w686 w691 w696 w702 w706 w711 w716 w721 w726 w731 w736 w741 w746 w752 w755 w760 w765 w770 w775 w780 w785 w790 w795 w800 w805 w810 w815 w820 w825 w830 w835 w840 w845 w850 w855 w860 w865 w870 w875 w880 w885 w890 w896]
      tunnel: w640 -> [w644 w649 w654 w659 w664 w669 w674 w679 w684 w689 w694 w699 w704 w709 w714 w719 w724 w729 w734 w739 w744 w749 w758 w763 w768 w773 w778 w783 w788 w793 w798 w803 w808 w813 w818 w823 w828 w833 w838 w843 w848 w853 w858 w863 w868 w873 w878 w883 w888 w893 _]
      tunnel: [w644 w649 w654 w659 w664 w669 w674 w679 w684 w689 w694 w699 w704 w709 w714 w719 w724 w729 w734 w739 w744 w749 w758 w763 w768 w773 w778 w783 w788 w793 w798 w803 w808 w813 w818 w823 w828 w833 w838 w843 w848 w853 w858 w863 w868 w873 w878 w883 w888 w893 TRUE] -> w639
      event "Open": Value Change {
        n284 = event-data() -> ()  [unwired: 1 in, 1 out]
        n285 = Enqueue Element(queue=w646, element=BiSS_Interface_Demo_Functions."Open" ("Events"), error in (no error)=w648) -> (error out=w647:errorcluster)  [unwired: 1 in, 2 out]
      }
      event "Close": Value Change {
        n286 = event-data() -> ()  [unwired: 1 in, 1 out]
        n287 = Enqueue Element(queue=w651, element=BiSS_Interface_Demo_Functions."Close" ("Events"), error in (no error)=w653) -> (error out=w652:errorcluster)  [unwired: 1 in, 2 out]
      }
      event "Set Interface": Value Change {
        n288 = event-data() -> ()  [unwired: 1 in, 1 out]
        n289 = Enqueue Element(queue=w656, element=BiSS_Interface_Demo_Functions."Set Interface" ("Events"), error in (no error)=w658) -> (error out=w657:errorcluster)  [unwired: 1 in, 2 out]
      }
      event "Get Interface": Value Change {
        n290 = event-data() -> ()  [unwired: 1 in, 1 out]
        n291 = Enqueue Element(queue=w661, element=BiSS_Interface_Demo_Functions."Get Interface" ("Events"), error in (no error)=w663) -> (error out=w662:errorcluster)  [unwired: 1 in, 2 out]
      }
      event "Get Interface Info": Value Change {
        n292 = event-data() -> ()  [unwired: 1 in, 1 out]
        n293 = Enqueue Element(queue=w666, element=BiSS_Interface_Demo_Functions."Get Interface Info" ("Events"), error in (no error)=w668) -> (error out=w667:errorcluster)  [unwired: 1 in, 2 out]
      }
      event "Auto Detection": Value Change {
        n294 = event-data() -> ()  [unwired: 1 in, 1 out]
        n295 = Enqueue Element(queue=w671, element=BiSS_Interface_Demo_Functions."Auto Detection" ("Events"), error in (no error)=w672) -> (error out=w673:errorcluster)  [unwired: 1 in, 2 out]
      }
      event "Set Com Param": Value Change {
        n296 = event-data() -> ()  [unwired: 1 in, 1 out]
        n297 = Enqueue Element(queue=w676, element=BiSS_Interface_Demo_Functions."Set Com Param" ("Events"), error in (no error)=w678) -> (error out=w677:errorcluster)  [unwired: 1 in, 2 out]
      }
      event "Get Com Param": Value Change {
        n298 = event-data() -> ()  [unwired: 1 in, 1 out]
        n299 = Enqueue Element(queue=w681, element=BiSS_Interface_Demo_Functions."Get Com Param" ("Events"), error in (no error)=w683) -> (error out=w682:errorcluster)  [unwired: 1 in, 2 out]
      }
      event "Set Frame Param": Value Change {
        n300 = event-data() -> ()  [unwired: 1 in, 1 out]
        n301 = Enqueue Element(queue=w686, element=BiSS_Interface_Demo_Functions."Set Frame Param" ("Events"), error in (no error)=w687) -> (error out=w688:errorcluster)  [unwired: 1 in, 2 out]
      }
      event "Get Frame Param": Value Change {
        n302 = event-data() -> ()  [unwired: 1 in, 1 out]
        n303 = Enqueue Element(queue=w691, element=BiSS_Interface_Demo_Functions."Get Frame Param" ("Events"), error in (no error)=w693) -> (error out=w692:errorcluster)  [unwired: 1 in, 2 out]
      }
      event "Write Master Params": Value Change {
        n304 = event-data() -> ()  [unwired: 1 in, 1 out]
        n305 = Enqueue Element(queue=w696, element=BiSS_Interface_Demo_Functions."Write Master Params" ("Events"), error in (no error)=w698) -> (error out=w697:errorcluster)  [unwired: 1 in, 2 out]
      }
      event "Set FTDI Freq": Value Change {
        n306 = event-data() -> ()  [unwired: 1 in, 1 out]
        n307 = Enqueue Element(queue=w702, element=BiSS_Interface_Demo_Functions."Set FTDI Freq" ("Events"), error in (no error)=w703) -> (error out=w700:errorcluster)  [unwired: 1 in, 2 out]
      }
      event "Init BiSS Comm": Value Change {
        n308 = event-data() -> ()  [unwired: 1 in, 1 out]
        n309 = Enqueue Element(queue=w706, element=BiSS_Interface_Demo_Functions."Init BiSS Comm" ("Events"), error in (no error)=w708) -> (error out=w707:errorcluster)  [unwired: 1 in, 2 out]
      }
      event "Write Slave Register": Value Change {
        n310 = event-data() -> ()  [unwired: 1 in, 1 out]
        n311 = Enqueue Element(queue=w711, element=BiSS_Interface_Demo_Functions."Write Slave Register" ("Events"), error in (no error)=w713) -> (error out=w712:errorcluster)  [unwired: 1 in, 2 out]
      }
      event "Read Slave Register": Value Change {
        n312 = event-data() -> ()  [unwired: 1 in, 1 out]
        n313 = Enqueue Element(queue=w716, element=BiSS_Interface_Demo_Functions."Read Slave Register" ("Events"), error in (no error)=w718) -> (error out=w717:errorcluster)  [unwired: 1 in, 2 out]
      }
      event "Read SCD": Value Change {
        n314 = event-data() -> ()  [unwired: 1 in, 1 out]
        n315 = Enqueue Element(queue=w721, element=BiSS_Interface_Demo_Functions."Read SCD" ("Events"), error in (no error)=w723) -> (error out=w722:errorcluster)  [unwired: 1 in, 2 out]
      }
      event "Send Command": Value Change {
        n316 = event-data() -> ()  [unwired: 1 in, 1 out]
        n317 = Enqueue Element(queue=w726, element=BiSS_Interface_Demo_Functions."Send Command" ("Events"), error in (no error)=w728) -> (error out=w727:errorcluster)  [unwired: 1 in, 2 out]
      }
      event "Set Slave Label": Value Change {
        n318 = event-data() -> ()  [unwired: 1 in, 1 out]
        n319 = Enqueue Element(queue=w731, element=BiSS_Interface_Demo_Functions."Set Slave Label" ("Events"), error in (no error)=w733) -> (error out=w732:errorcluster)  [unwired: 1 in, 2 out]
      }
      event "Get Slave Label": Value Change {
        n320 = event-data() -> ()  [unwired: 1 in, 1 out]
        n321 = Enqueue Element(queue=w736, element=BiSS_Interface_Demo_Functions."Get Slave Label" ("Events"), error in (no error)=w738) -> (error out=w737:errorcluster)  [unwired: 1 in, 2 out]
      }
      event "Set SCD Content Labels": Value Change {
        n322 = event-data() -> ()  [unwired: 1 in, 1 out]
        n323 = Enqueue Element(queue=w741, element=BiSS_Interface_Demo_Functions."Set SCD Content Labels" ("Events"), error in (no error)=w743) -> (error out=w742:errorcluster)  [unwired: 1 in, 2 out]
      }
      event "Get SCD Content Labels": Value Change {
        n324 = event-data() -> ()  [unwired: 1 in, 1 out]
        n325 = Enqueue Element(queue=w746, element=BiSS_Interface_Demo_Functions."Get SCD Content Labels" ("Events"), error in (no error)=w748) -> (error out=w747:errorcluster)  [unwired: 1 in, 2 out]
      }
      event "Get SCD Content": Value Change {
        n326 = event-data() -> ()  [unwired: 1 in, 1 out]
        n327 = Enqueue Element(queue=w752, element=BiSS_Interface_Demo_Functions."Get SCD Content" ("Events"), error in (no error)=w753) -> (error out=w751:errorcluster)  [unwired: 1 in, 2 out]
      }
      event "Get SCD Content Ex": Value Change {
        n328 = event-data() -> ()  [unwired: 1 in, 1 out]
        n329 = Enqueue Element(queue=w755, element=BiSS_Interface_Demo_Functions."Get SCD Content Ex" ("Events"), error in (no error)=w756) -> (error out=w754:errorcluster)  [unwired: 1 in, 2 out]
      }
      event "Set SCD Content Params": Value Change {
        n330 = event-data() -> ()  [unwired: 1 in, 1 out]
        n331 = Enqueue Element(queue=w760, element=BiSS_Interface_Demo_Functions."Set SCD Content Params" ("Events"), error in (no error)=w761) -> (error out=w759:errorcluster)  [unwired: 1 in, 2 out]
      }
      event "Get SCD Content Params": Value Change {
        n332 = event-data() -> ()  [unwired: 1 in, 1 out]
        n333 = Enqueue Element(queue=w765, element=BiSS_Interface_Demo_Functions."Get SCD Content Params" ("Events"), error in (no error)=w766) -> (error out=w764:errorcluster)  [unwired: 1 in, 2 out]
      }
      event "Read SCD Frames": Value Change {
        n334 = event-data() -> ()  [unwired: 1 in, 1 out]
        n335 = Enqueue Element(queue=w770, element=BiSS_Interface_Demo_Functions."Read SCD Frames" ("Events"), error in (no error)=w771) -> (error out=w769:errorcluster)  [unwired: 1 in, 2 out]
      }
      event "Get SCD Frame": Value Change {
        n336 = event-data() -> ()  [unwired: 1 in, 1 out]
        n337 = Enqueue Element(queue=w775, element=BiSS_Interface_Demo_Functions."Get SCD Frame" ("Events"), error in (no error)=w776) -> (error out=w774:errorcluster)  [unwired: 1 in, 2 out]
      }
      event "Get SCD Frame Ex": Value Change {
        n338 = event-data() -> ()  [unwired: 1 in, 1 out]
        n339 = Enqueue Element(queue=w780, element=BiSS_Interface_Demo_Functions."Get SCD Frame Ex" ("Events"), error in (no error)=w781) -> (error out=w779:errorcluster)  [unwired: 1 in, 2 out]
      }
      event "Get SCD Frame Content": Value Change {
        n340 = event-data() -> ()  [unwired: 1 in, 1 out]
        n341 = Enqueue Element(queue=w785, element=BiSS_Interface_Demo_Functions."Get SCD Frame Content" ("Events"), error in (no error)=w786) -> (error out=w784:errorcluster)  [unwired: 1 in, 2 out]
      }
      event "Get SCD Frame Content Ex": Value Change {
        n342 = event-data() -> ()  [unwired: 1 in, 1 out]
        n343 = Enqueue Element(queue=w790, element=BiSS_Interface_Demo_Functions."Get SCD Frame Content Ex", error in (no error)=w792) -> (error out=w791:errorcluster)  [unwired: 1 in, 2 out]
      }
      event "Get EDS Param": Value Change {
        n344 = event-data() -> ()  [unwired: 1 in, 1 out]
        n345 = Enqueue Element(queue=w795, element=BiSS_Interface_Demo_Functions."Get EDS Param" ("Events"), error in (no error)=w796) -> (error out=w794:errorcluster)  [unwired: 1 in, 2 out]
      }
      event "Set EDS Param": Value Change {
        n346 = event-data() -> ()  [unwired: 1 in, 1 out]
        n347 = Enqueue Element(queue=w800, element=BiSS_Interface_Demo_Functions."Set EDS Param" ("Events"), error in (no error)=w801) -> (error out=w799:errorcluster)  [unwired: 1 in, 2 out]
      }
      event "Set EDS Register": Value Change {
        n348 = event-data() -> ()  [unwired: 1 in, 1 out]
        n349 = Enqueue Element(queue=w805, element=BiSS_Interface_Demo_Functions."Set EDS Register" ("Events"), error in (no error)=w806) -> (error out=w804:errorcluster)  [unwired: 1 in, 2 out]
      }
      event "Get EDS Register": Value Change {
        n350 = event-data() -> ()  [unwired: 1 in, 1 out]
        n351 = Enqueue Element(queue=w810, element=BiSS_Interface_Demo_Functions."Get EDS Register" ("Events"), error in (no error)=w811) -> (error out=w809:errorcluster)  [unwired: 1 in, 2 out]
      }
      event "Read EDS Params": Value Change {
        n352 = event-data() -> ()  [unwired: 1 in, 1 out]
        n353 = Enqueue Element(queue=w815, element=BiSS_Interface_Demo_Functions."Read EDS Params" ("Events"), error in (no error)=w816) -> (error out=w814:errorcluster)  [unwired: 1 in, 2 out]
      }
      event "Write EDS Params": Value Change {
        n354 = event-data() -> ()  [unwired: 1 in, 1 out]
        n355 = Enqueue Element(queue=w820, element=BiSS_Interface_Demo_Functions."Write EDS Params" ("Events"), error in (no error)=w821) -> (error out=w819:errorcluster)  [unwired: 1 in, 2 out]
      }
      event "Get DLL Version": Value Change {
        n356 = event-data() -> ()  [unwired: 1 in, 1 out]
        n357 = Enqueue Element(queue=w825, element=BiSS_Interface_Demo_Functions."Get DLL Version" ("Events"), error in (no error)=w826) -> (error out=w824:errorcluster)  [unwired: 1 in, 2 out]
      }
      event "Calculate CRC": Value Change {
        n358 = event-data() -> ()  [unwired: 1 in, 1 out]
        n359 = Enqueue Element(queue=w830, element=BiSS_Interface_Demo_Functions."Calculate CRC" ("Events"), error in (no error)=w831) -> (error out=w829:errorcluster)  [unwired: 1 in, 2 out]
      }
      event "Calculate CRC Ex": Value Change {
        n360 = event-data() -> ()  [unwired: 1 in, 1 out]
        n361 = Enqueue Element(queue=w835, element=BiSS_Interface_Demo_Functions."Calculate CRC Ex" ("Events"), error in (no error)=w836) -> (error out=w834:errorcluster)  [unwired: 1 in, 2 out]
      }
      event "Save DLL Config": Value Change {
        n362 = event-data() -> ()  [unwired: 1 in, 1 out]
        n363 = Enqueue Element(queue=w840, element=BiSS_Interface_Demo_Functions."Save DLL Config" ("Events"), error in (no error)=w841) -> (error out=w839:errorcluster)  [unwired: 1 in, 2 out]
      }
      event "Load DLL Config": Value Change {
        n364 = event-data() -> ()  [unwired: 1 in, 1 out]
        n365 = Enqueue Element(queue=w845, element=BiSS_Interface_Demo_Functions."Load DLL Config" ("Events"), error in (no error)=w846) -> (error out=w844:errorcluster)  [unwired: 1 in, 2 out]
      }
      event "Get Last Error": Value Change {
        n366 = event-data() -> ()  [unwired: 1 in, 1 out]
        n367 = Enqueue Element(queue=w850, element=BiSS_Interface_Demo_Functions."Get Last Error" ("Events"), error in (no error)=w851) -> (error out=w849:errorcluster)  [unwired: 1 in, 2 out]
      }
      event "Get MB3U Pins": Value Change {
        n368 = event-data() -> ()  [unwired: 1 in, 1 out]
        n369 = Enqueue Element(queue=w855, element=BiSS_Interface_Demo_Functions."Get MB3U Pins" ("Events"), error in (no error)=w856) -> (error out=w854:errorcluster)  [unwired: 1 in, 2 out]
      }
      event "Set MB3U Pins": Value Change {
        n370 = event-data() -> ()  [unwired: 1 in, 1 out]
        n371 = Enqueue Element(queue=w860, element=BiSS_Interface_Demo_Functions."Set MB3U Pins" ("Events"), error in (no error)=w861) -> (error out=w859:errorcluster)  [unwired: 1 in, 2 out]
      }
      event "Write Master Register": Value Change {
        n372 = event-data() -> ()  [unwired: 1 in, 1 out]
        n373 = Enqueue Element(queue=w865, element=BiSS_Interface_Demo_Functions."Write Master Register" ("Events"), error in (no error)=w866) -> (error out=w864:errorcluster)  [unwired: 1 in, 2 out]
      }
      event "Read Master Register": Value Change {
        n374 = event-data() -> ()  [unwired: 1 in, 1 out]
        n375 = Enqueue Element(queue=w870, element=BiSS_Interface_Demo_Functions."Read Master Register" ("Events"), error in (no error)=w871) -> (error out=w869:errorcluster)  [unwired: 1 in, 2 out]
      }
      event "Get Master Register": Value Change {
        n376 = event-data() -> ()  [unwired: 1 in, 1 out]
        n377 = Enqueue Element(queue=w875, element=BiSS_Interface_Demo_Functions."Get Master Register" ("Events"), error in (no error)=w876) -> (error out=w874:errorcluster)  [unwired: 1 in, 2 out]
      }
      event "Save Master Config": Value Change {
        n378 = event-data() -> ()  [unwired: 1 in, 1 out]
        n379 = Enqueue Element(queue=w880, element=BiSS_Interface_Demo_Functions."Save Master Config" ("Events"), error in (no error)=w881) -> (error out=w879:errorcluster)  [unwired: 1 in, 2 out]
      }
      event "Save Register": Value Change {
        n380 = event-data() -> ()  [unwired: 1 in, 1 out]
        n381 = Enqueue Element(queue=w885, element=BiSS_Interface_Demo_Functions."Save Register" ("Events"), error in (no error)=w886) -> (error out=w884:errorcluster)  [unwired: 1 in, 2 out]
      }
      event "Load Register": Value Change {
        n382 = event-data() -> ()  [unwired: 1 in, 1 out]
        n383 = Enqueue Element(queue=w890, element=BiSS_Interface_Demo_Functions."Load Register" ("Events"), error in (no error)=w891) -> (error out=w889:errorcluster)  [unwired: 1 in, 2 out]
      }
      event "Stop Button": Value Change {
        n384 = event-data() -> ()  [unwired: 1 in, 1 out]
        n385 = Enqueue Element At Opposite End(queue=w896, element=BiSS_Interface_Demo_Functions."Stop Demo" ("Events"), error in (no error)=w897) -> (error out=w895:errorcluster)  [unwired: 1 in, 2 out]
      }
    }
    n386 = call <vilib>:"Simple Error Handler.vi"("error in (no error)"=w641) -> ()  [unwired: 4 in, 5 out]
  }
